vi "rio_veloster8.vi"() -> ()   [LabVIEW 2012]
uses:
  <vilib>/xnet/xnet.llb/XNET Frame CAN.ctl
  <vilib>/xnet/xnet.llb/XNET Frame Type CAN.ctl
  G_rio.vi
  <vilib>/FPGAPlugInAG/cRIO-9113/niLvFpga_Open_cRIO-9113.vi
  <vilib>/rvi/interface/common/dynamic/niFpgaDynamicAddResources.vi
  <vilib>/FPGAPlugInAG/Dynamic/niLvFpga_Abort_Dynamic.vi
  <vilib>/FPGAPlugInAG/Dynamic/niLvFpga_Run_Dynamic.vi
  <vilib>/Utility/error.llb/Error Cluster From Error Code.vi
  <vilib>/Instr/_visa.llb/VISA Configure Serial Port (Instr).vi
  <vilib>/xnet/xnet.llb/XNET Create Session (Frame Output Stream).vi
  <vilib>/xnet/xnet.llb/XNET Create Session (Frame Input Stream).vi
  <vilib>/xnet/xnet.llb/XNET Read (Frame CAN).vi
  <vilib>/rvi/errors/niLvFpgaAdjustHostInterfaceError.vi
  <vilib>/xnet/xnet.llb/XNET Write (Frame CAN).vi
  <vilib>/Analysis/Matrix/Numeric/Conversions/Array To Matrix - RA2.vi
  <vilib>/Analysis/Matrix/Numeric/Multiply/Multiply - RM,RM.vi
  <vilib>/Analysis/Matrix/Numeric/Add/Add - RM,RM.vi
  <vilib>/Analysis/baseanly.llb/Real Inverse Matrix.vi
  <vilib>/Analysis/Matrix/Numeric/Subtract/Subtract - RM,RM.vi
  <vilib>/Analysis/Matrix/Numeric/Conversions/Array To Matrix - RA.vi
  <vilib>/Analysis/Matrix/Numeric/Multiply/Multiply - R,RM.vi
  <vilib>/Analysis/Matrix/Numeric/Conversions/Matrix To Array - RM.vi
  <vilib>/rvi/interface/nirviOpenFPGA/nirviOpenFPGA.xnode
  FPGA Bitfiles/autonomous_FPGATarget2_fpga3_8ngZXtRRx8Y.lvbitx
  fpga/fpga3.vi
  <vilib>/rvi/interface/nirviMethod/nirviMethod.xnode
  <vilib>/rvi/interface/nirviReadWriteControl/nirviReadWriteControl.xnode
  <vilib>/rvi/interface/Simulation/niFpgaSimulationCallBeginRW.vi
  <vilib>/FPGAPlugInAG/Dynamic/niLvFpga_StartFifo_Dynamic.vi
  <vilib>/rvi/errors/niLvFpgaMergeErrorWithErrorCode.vi
  <resource>/objmgr/xnet.rc
  NiFpgaLv.dll
  <vilib>/FPGAPlugInAG/Dynamic/niLvFpga_ReadFifo_Dynamic.vi
  <vilib>/Analysis/Matrix/NI_Matrix.lvlib
  <vilib>/Analysis/NI_AALBase.lvlib
panel:
  out "Pos_time 10":i32
  out "FPGA VI Reference Out":refnum<k20>
  out "T PWM":u16
  out "B PWM":u16
  out "solenoid":bool
  out "brk enc":u8
  out "shift lever":dbl
  in  "LCM":bool=TRUE
  out "mobileye":u8[](array[numeric])
  out "timer":u32
  out "Mobileye_time 100":u32
  out "H_GPS":dbl
  out "pos":dbl[](array[numeric])
  out "gps pos error":dbl
  in  "GPS init":bool=TRUE
  out "battery voltage":dbl
  in  "Gear Manual":i32(slide)=1 scale=-1.0..1.0
  out "map":i32=2
  out "P, R, D":i32
  out "kalman heading error":dbl
  out "Kalman init":bool
  out "VS_CAN":dbl
  in  "brake":bool
  in  "Slide":dbl(slide) min=-50.0 max=50.0 step=50.0 scale=-50.0..50.0
  out "novatel":refnum<visa-resource-name>
  in  "ublox":bool=TRUE
  out "rest":u8[](array[numeric])
  out "GPS_novatel_time":u32
  out "GPS_Ublox_time 100":u32
  out "Con_time 10":i32
  out "CAN_time 10":u32
  out "gps2":refnum<visa-resource-name>
  out "gps1":refnum<visa-resource-name>
  out "Heading":dbl
  out "ecef ref":dbl[](array[numeric])
  out "h_gps":dbl
  out "pos_gps":dbl[](array[numeric]) format="%#_19f"
  out "get heading":bool
  out "get position":bool
  out "dt":dbl
  out "rt":dbl
  out "CAN Comm Enabled":bool
  in  "SPAS Enable":bool=TRUE
  in  "file write":bool
  out "data write":refnum<file>
  out "file rw error":errorcluster
  out "car can error":errorcluster
  out "CAN write":refnum<k21>
  out "CAN read":refnum<k21>
  out "Ref steer":dbl=1.0
  in  "Steer input":bool=TRUE
  in  "Ref steer manual":dbl(knob) scale=-550.0..550.0
  out "Ref vel":dbl=1.0
  in  "Ref vel manual":dbl
  in  "Velocity input":bool
  out "Auto":bool
  out "Run":bool
  out "E - STOP":bool
  out "Throttle Enable":bool=TRUE
  # "P"
  # "R"
  # "D"
  # "Ref steer manual"
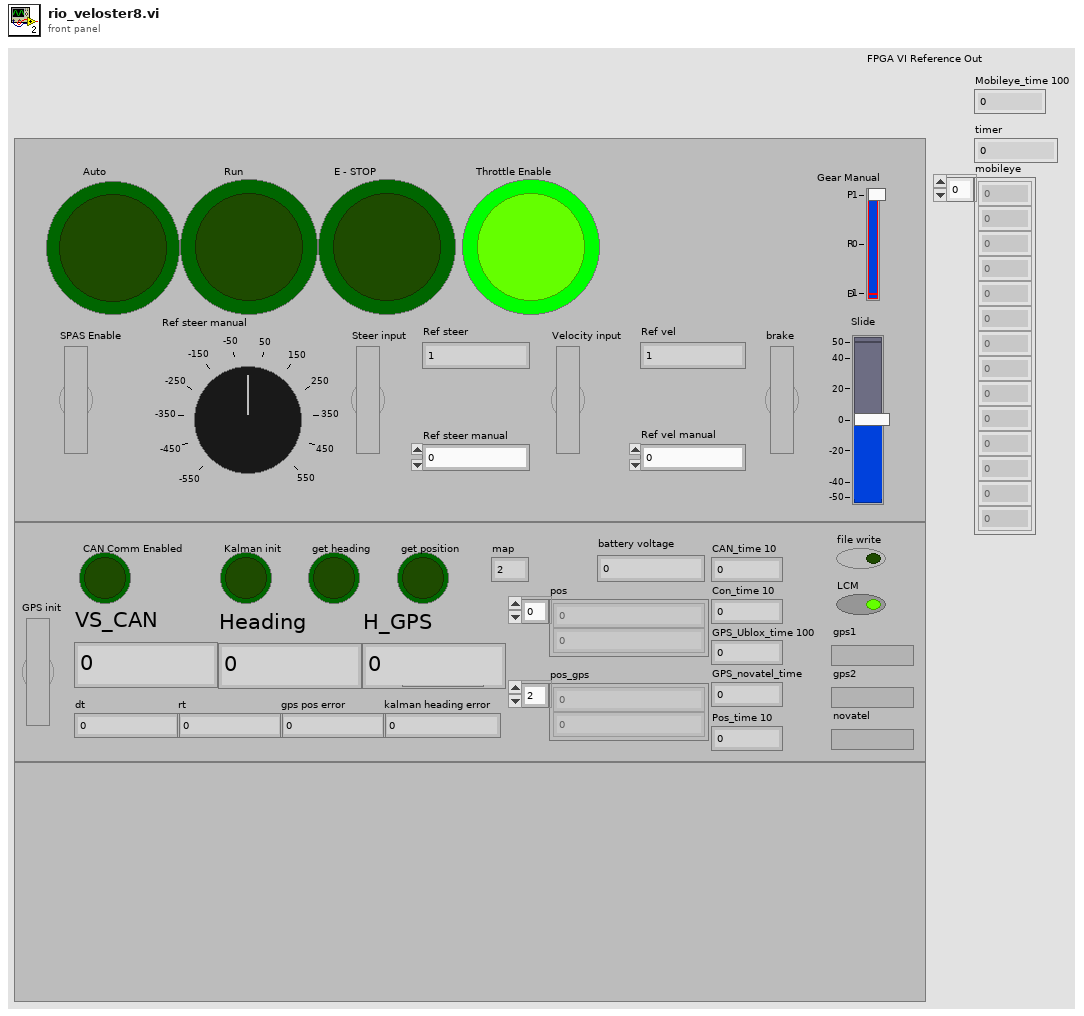
[diagram p1: front panel]
types:
  T1 = enum16{"open", "replace", "create", "open or create", "replace or create", "replace or create with confirmation"}
  T2 = typedef "XNET Frame CAN.ctl" = cluster{"timestamp":timestamp, "payload":u8[], "identifier":u32, "type":T3, "extended?":bool, "echo?":bool}
  T3 = typedef "XNET Frame Type CAN.ctl" = u8
  T4 = cluster{"connection ID":refnum<k16>, "net address":u32, "port":u16}
  T5 = cluster{"hash":i64, "sys time":i64, "mobileye":u8[]}
  T6 = cluster{"hash":i64, "sys time":i64, "time":dbl, "yaw_rate":dbl, "mdps torque":dbl, "mdps str_ang":dbl, "VS_CAN":dbl, "lat_accel":dbl, "mcp":dbl, "accel pedal value":dbl, "tps":dbl, "odometer":dbl, "battery voltage":dbl, "WHL_SPD_RR":dbl, "WHL_SPD_RL":dbl, "WHL_SPD_FR":dbl, "WHL_SPD_FL":dbl}
  T7 = cluster{"LCC[0]":dbl, "LCC[1]":dbl, "LCC[2]":dbl, "LCC[3]":dbl, "LCC[4]":dbl, "LCC[5]":dbl, "LCC[6]":dbl, "LCC[7]":dbl, "LCC[8]":dbl, "LCC[9]":dbl, "LCC[10]":dbl, "LCC[11]":dbl, "LCC[12]":dbl, "LCC[13]":dbl, "LCC[14]":dbl}
  T8 = cluster{"hash":i64, "sys time":i64, "time":dbl, "x":dbl, "y":dbl, "h":dbl, "numSV":i32, "postype":i32, "lag":i32, "hordev":dbl, "lat":dbl, "lon":dbl, "hgt":dbl, "map_idx":i32}
  T9 = cluster{"vel[0]":dbl, "vel[1]":dbl, "vel[2]":dbl, "vel[3]":dbl, "vel[4]":dbl, "vel[5]":dbl, "vel[6]":dbl}
  T10 = cluster{"hash":i64, "sys time":i64, "time":dbl, "speed":dbl, "heading":dbl, "lat":dbl, "lon":dbl}
  T11 = cluster{"output[0]":dbl, "output[1]":dbl, "output[2]":dbl, "output[3]":dbl, "output[4]":dbl, "output[5]":dbl, "output[6]":dbl, "output[7]":dbl, "output[8]":dbl, "output[9]":dbl, "output[10]":dbl, "output[11]":dbl, "output[12]":dbl, "output[13]":dbl, "output[14]":dbl}
  T12 = cluster{"output[0]":dbl, "output[1]":dbl, "output[2]":dbl, "output[3]":dbl, "output[4]":dbl, "output[5]":dbl, "output[6]":dbl}
  T13 = typedef "NI_Matrix.lvlib/RealMatrix.ctl" = dbl[][]
  T14 = cluster{"Real 2D Array[0]":dbl, "Real 2D Array[1]":dbl, "Real 2D Array[2]":dbl, "Real 2D Array[3]":dbl, "Real 2D Array[4]":dbl}
  T15 = cluster{"hash":i64, "sys time":i64, "dt":dbl, "x":dbl, "y":dbl, "speed":dbl, "heading":dbl, "yaw_rate":dbl}
  T16 = cluster{"hash":i64, "sys time":i64, "ref_vel":dbl, "ref_steer":dbl}
  T17 = cluster{"hash":i64, "sys time":i64, "Auto":bool, "Run":bool, "Solenoid":bool, "T lim":bool, "brk_enc":u8, "B PWM":u16, "T PWM":u16, "ref_vel":dbl, "ref_bkr_enc":dbl, "ref_apv":dbl, "ref_steer":dbl}
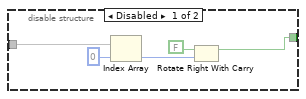
[diagram p5: hidden frame]
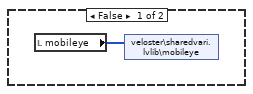
[diagram p7: hidden frame]
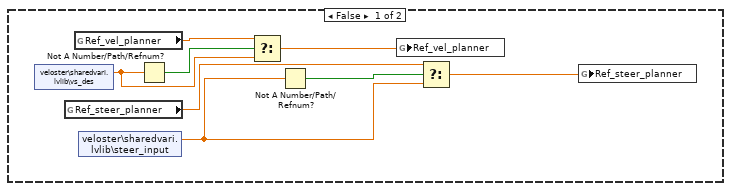
[diagram p9: hidden frame]
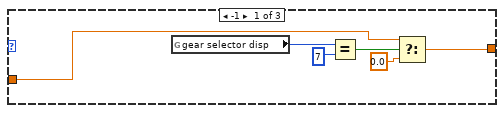
[diagram p14: hidden frame]
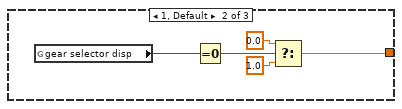
[diagram p18: hidden frame]
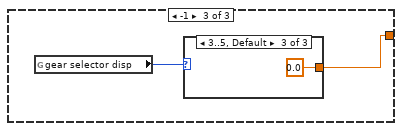
[diagram p19: hidden frame]
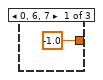
[diagram p20: hidden frame]
diagram:
  n1 = flat-sequence {
    frame #0 {
      w3 = FALSE ("GPS init")
      w2 = 0.0 ("Ref_vel_planner")
      n2 = xnode "Open FPGA VI Reference"() -> ("FPGA VI Reference Out"=w12:refnum<k20>, "error out"=w11:errorcluster)  [unwired: 2 in]
      n3 = global write "G_rio.vi" "Ref_steer_planner"(w2) -> ()
      n4 = global write "G_rio.vi" "Ref_vel_planner"(w2) -> ()
      n5 = local write "rest"(u8[] [] ("rest")) -> ()
      n6 = local write "brake"(w3) -> ()
      n7 = local write "GPS init"(w3) -> ()
      n8 = local write "Velocity input"(w3) -> ()
      n9 = xnode "Invoke Method"("FPGA VI Reference In"=w12, "error in"=w11) -> ("FPGA VI Reference Out"=w10:refnum<k20>, "error out"=w9:errorcluster)
      n10 = xnode "Invoke Method"("FPGA VI Reference In"=w10, "error in"=w9, "Wait Until Done (F)"=FALSE) -> ("FPGA VI Reference Out"=w8:refnum<k20>, "error out"=w7:errorcluster)
      n11 = xnode "Invoke Method"("FPGA VI Reference In"=w8, "error in"=w7) -> ("FPGA VI Reference Out"=w6:refnum<k20>, "error out"=w5:errorcluster)
      n12 = xnode "Invoke Method"("FPGA VI Reference In"=w6, "error in"=w5) -> ("FPGA VI Reference Out"=→"FPGA VI Reference Out":refnum<k20>)  [unwired: 1 out]
    }
    frame #1 {
      n13 = flat-sequence {
        frame #0 {
          w61 = 9 ("map")
          n14 = global write "G_rio.vi" "T lim counter 2"(u16 300 ("T lim counter 2")) -> ()
          n15 = local write "rest"(u8[] [] ("rest")) -> ()
          n16 = call "getecefdcmref.vi"("map"=w61) -> ("XYZ"=→"ecef ref":dbl[])  [unwired: 10 in, 4 out]
          "Kalman init" <- TRUE ("pos linit")
          "map" <- w61
        }
      }
      n17 = disable-structure shown="Enabled" {
        frame Enabled {
          n18 = call-poly "VISA Configure Serial Port"("VISA resource name"=refnum<visa-resource-name> "ASRL1::INSTR", "timeout (10sec)"=u32 10, "baud rate (9600)"=u32 9600) -> ("VISA resource name out"=→"novatel":refnum<visa-resource-name>)  [unwired: 11 in, 1 out]
          n19 = call-poly "VISA Configure Serial Port"("VISA resource name"=refnum<visa-resource-name> "USB0::0x1546::0x01A6::NI-VISA-1::1::RAW", "timeout (10sec)"=u32 1, "baud rate (9600)"=u32 115200) -> ("VISA resource name out"=→"gps1":refnum<visa-resource-name>)  [unwired: 11 in, 1 out]
          n20 = call-poly "VISA Configure Serial Port"("VISA resource name"=refnum<visa-resource-name> "USB0::0x1546::0x01A6::NI-VISA-0::1::RAW", "timeout (10sec)"=u32 1, "baud rate (9600)"=u32 115200) -> ("VISA resource name out"=→"gps2":refnum<visa-resource-name>)  [unwired: 11 in, 1 out]
        }
        frame Disabled {
        }
      }
      n21 = flat-sequence {
        frame #0 {
          n22 = property class="XNET System"() -> (error out=w28:errorcluster, "Devices"=w42:refnum<k21>[])  [unwired: 2 in, 1 out]
          n23 = Index Array(array=w42, index=0) -> (element=w40:refnum<k21>)
          n24 = property class="XNET Device"(reference=w40, error in=w28) -> (error out=→"car can error":errorcluster, "Intfs"=w39:refnum<k21>[])  [unwired: 1 out]
          n25 = Index Array(array=w39, index=0) -> (element=w30:refnum<k21>)
          n26 = call-poly <vilib>:"XNET Create Session.vi"("cluster (:memory:)"=refnum<k21> "nixnet_example.CAN_Cluster", "interface"=w30) -> ("session out"=w31:refnum<k21>)  [unwired: 1 in, 12 out]
          n27 = call-poly <vilib>:"XNET Create Session.vi"("cluster (:memory:)"=refnum<k21> "nixnet_example.CAN_Cluster", "interface"=w30) -> ("session out"=w37:refnum<k21>)  [unwired: 1 in, 12 out]
          n28 = property class="XNET Session"(reference=w31, "Intf.BaudRate"=u32 500000 ("Interface:Baud Rate")) -> (reference out=w33:refnum<k21>)  [unwired: 1 in, 1 out]
          n29 = property class="XNET Session"(reference=w37, "Intf.BaudRate"=u32 500000 ("Interface:Baud Rate")) -> (reference out=w35:refnum<k21>)  [unwired: 1 in, 1 out]
          n30 = call <vilib>:"XNET Start.vi"("session in"=w33) -> ("session out"=→"CAN read":refnum<k21>)  [unwired: 1 in, 13 out]
          n31 = call <vilib>:"XNET Start.vi"("session in"=w35) -> ("session out"=→"CAN write":refnum<k21>)  [unwired: 1 in, 13 out]
        }
      }
      n32 = case shown="True" "file write" {
        frame False {
        }
        frame True {
          n33 = Open/Create/Replace File(file path (use dialog)=path "c:/datasave", operation (0:open)=T1."replace or create", access (0:read/write)=enum16{"read/write", "read-only", "write-only"}."write-only") -> (refnum out=→"data write":refnum<file>, cancelled=w65:bool, error out=→"file rw error":errorcluster)  [unwired: 3 in]
          n34 = Not(x=w65) -> (.not. x?=w64:bool)
          n35 = local write "file write"(w64) -> ()
        }
      }
      n36 = case shown="True" TRUE {
        frame False {
        }
        frame True {
          n37 = flat-sequence {
            frame #0 {
              w22 = u16 7667 ("port")
              n38 = Decrement(x=w22) -> (x-1=w21:u16)
              n39 = UDP Open(11:w21) -> (port=w24:refnum<k16>)  [unwired: 4 in, 2 out]
              n40 = global read "G_rio.vi" "LCM"() -> (w26:T4)
              n41 = Bundle By Name(cluster=w26, "port"=w22, "connection ID"=w24, "net address"=u32 4294967295) -> (w25:T4)
              n42 = global write "G_rio.vi" "LCM"(w25) -> ()
            }
          }
          n43 = flat-sequence {
            frame #0 {
              w16 = u16 7668 ("port")
              n44 = global read "G_rio.vi" "LCM PC"() -> (w20:T4)
              n45 = UDP Open(11:w16) -> (port=w18:refnum<k16>)  [unwired: 4 in, 2 out]
              n46 = Bundle By Name(cluster=w20, "port"=w16, "connection ID"=w18, "net address"=u32 0) -> (w19:T4)
              n47 = global write "G_rio.vi" "LCM PC"(w19) -> ()
            }
          }
        }
      }
    }
    frame #2 {
      (unwired) FALSE
      n48 = disable-structure shown="Enabled" {
        frame Enabled {
          n49 = while {
            stop <- FALSE stop-if-true
            n50 = flat-sequence {
              frame #0 {
                n51 = Wait Until Next ms Multiple(millisecond multiple=u32 100) -> (millisecond timer value=w71:u32)
                n52 = flat-sequence {
                  tunnel: w71 -> [w73]
                  frame #0 {
                    n53 = feedback #1(w73) -> (w74:u32)
                    n54 = feedback-in #1(w73) -> ()
                    n55 = Subtract(x=w73, y=w74) -> (x-y=→"Mobileye_time 100":u32)
                  }
                }
              }
              frame #1 {
                n56 = local read "FPGA VI Reference Out"() -> (w120:refnum<k20>)
                n57 = xnode "Read/Write Control"("FPGA VI Reference In"=w120) -> ("m 700"=w80:u8[], "m 760"=w116:u8[], "m 710"=w105:u8[], "m 711"=w101:u8[], "m 720"=w99:u8[], "m 721"=w98:u8[], "m 722"=w97:u8[], "m 723"=w96:u8[], "m 724"=w95:u8[], "m 725"=w94:u8[], "m 726"=w93:u8[], "m 727"=w92:u8[], "m 728"=w91:u8[], "m 729"=w90:u8[])  [unwired: 1 in, 2 out]
                n58 = Build Array(w99, w98, w97, w96, w95, w94, w93, w92, w91, w90) -> (w89:u8[][])
                n59 = Index Array(array=w80, index #1=4 ("index"), index #4=8 ("index"), index #5=11 ("index")) -> (element #1=w113:u8, element #2=w112:u8, element #3=w111:u8, element #4=w110:u8, element #5=w109:u8)  [unwired: 2 in]
                n60 = Array Subset(array=w80, index=0, length=4) -> (w77:u8[])
                n61 = Array Subset(array=w116, index=4, length=3) -> (w108:u8[])
                n62 = Array Subset(array=w105, index=5, length=7) -> (w104:u8[])
                n63 = Array Subset(array=w101, index=6, length=6) -> (w100:u8[])
                n64 = Index Array(array=w77, index #1=0 ("index")) -> (element #1=w86:u8, element #2=w85:u8, element #3=w84:u8, element #4=w83:u8)  [unwired: 3 in]
                n65 = Build Array (concatenate)(w77, w113, w112, w111, w110, w109, w108, w104, w100) -> (w88:u8[])
                n66 = Join Numbers(hi=w86, lo=w85) -> ((hi.lo)=w82:u16)
                n67 = Join Numbers(hi=w84, lo=w83) -> ((hi.lo)=w81:u16)
                n68 = for {
                  tunnel: w89 -> [w122] mode=indexing
                  shift-right: [w125] -> w75
                  shift-left: w88 -> [w126]
                  n69 = Array Subset(array=w122, index=4, length=8) -> (w121:u8[])
                  n70 = disable-structure shown="Enabled" {
                    disable-tunnel: [w129 TRUE ("lsb carry out")] -> w127
                    disable-tunnel: w121 -> [w128 _]
                    frame Disabled {
                      n71 = Index Array(array=w128, index=0) -> (element=w131:u8)
                      n72 = Rotate Right With Carry(2:w131, 3:FALSE ("carry")) -> (1:w129:bool)  [unwired: 1 out]
                    }
                    frame Enabled {
                    }
                  }
                  n73 = case shown="True" w127 {
                    tunnel: w126 -> [w134 w137]
                    tunnel: [w134 w136] -> w125
                    tunnel: w121 -> [_ w135]
                    frame False {
                    }
                    frame True {
                      n74 = Build Array (concatenate)(w137, w135) -> (w136:u8[])
                    }
                  }
                }
                "mobileye" <- w75
                n75 = Join Numbers(hi=w82, lo=w81) -> ((hi.lo)=→"timer":u32)
              }
              frame #2 {
                n76 = local read "LCM"() -> (w138:bool)
                n77 = case shown="True" w138 {
                  frame False {
                    n78 = local read "mobileye"() -> (w139:u8[])
                    n79 = shared-variable "veloster\\sharedvari.lvlib\\mobileye"(w139) -> ()  [unwired: 1 in, 1 out]
                  }
                  frame True {
                    n80 = Get Date/Time In Seconds() -> (seconds since 1Jan1904=w144:timestamp)
                    n81 = local read "mobileye"() -> (w145:u8[])
                    n82 = To Double Precision Float(number=w144) -> (double precision float=w143:dbl)
                    n83 = global read "G_rio.vi" "LCM_EYE_RAW_T"() -> (w153:T5)
                    n84 = Unbundle By Name(w153) -> ("hash"=w152:i64)
                    n85 = Multiply(x=w143, y=1000000.0) -> (x*y=w141:dbl)
                    n86 = To Quad Integer(1:w141) -> (0:w140:i64)
                    n87 = call "hash.vi"("input"=w152) -> ("output"=w151:i64)  [unwired: 10 in]
                    n88 = Bundle By Name(cluster=w153, "hash"=w151, "sys time"=w140, "mobileye"=w145) -> (w150:T5)
                    n89 = Flatten To String(anything=w150, prepend array or string size? (T)=FALSE) -> (data string=w148:string)  [unwired: 2 in, 2 out]
                    n90 = global read "G_rio.vi" "LCM"() -> (w149:T4)
                    n91 = call "LCM_send.vi"("DATA"=w148, "ID"="EYE_RAW_T", "LCM"=w149) -> ()  [unwired: 6 in, 3 out]
                  }
                }
              }
            }
          }
        }
        frame Disabled {
        }
      }
      n92 = while {
        stop <- FALSE stop-if-true
        n93 = flat-sequence {
          frame #0 {
            n94 = Wait Until Next ms Multiple(millisecond multiple=u32 10) -> (millisecond timer value=w1396:u32)
            n95 = flat-sequence {
              tunnel: w1396 -> [w1399]
              frame #0 {
                n96 = feedback #2(w1399) -> (w1400:u32)
                n97 = feedback-in #2(w1399) -> ()
                n98 = Subtract(x=w1399, y=w1400) -> (x-y=→"CAN_time 10":u32)
              }
            }
          }
          frame #1 {
            n99 = local read "CAN read"() -> (w1404:refnum<k21>)
            n100 = call-poly <vilib>:"XNET Read.vi"("session in"=w1404) -> ("data"=w1403:T2[])  [unwired: 3 in, 11 out]
            n101 = Empty Array?(array=w1403) -> (empty?=w1402:bool)
            n102 = for {
              tunnel: w1403 -> [w1406] mode=indexing
              n103 = Unbundle By Name(w1406) -> ("timestamp"=w1405:timestamp, "identifier"=w1408:u32, "payload"=w1407:u8[])
              n104 = case shown="220" w1408 {
                tunnel: w1407 -> [_ w1443 w1478 w1497 w1538 w1569 w1601 w1608]
                tunnel: w1405 -> [_ w1438 _ _ _ _ _ _]
                frame 0, Default {
                }
                frame 544 {
                  w1412 = u16 8191
                  w1419 = u16 2047
                  n105 = global write "G_rio.vi" "timestamp"(w1438) -> ()
                  n106 = Index Array(array=w1443, index #1=5 ("index"), index #2=4 ("index"), index #3=1 ("index"), index #4=0 ("index"), index #5=7 ("index"), index #6=6 ("index")) -> (element #1=w1435:u8, element #2=w1434:u8, element #3=w1433:u8, element #4=w1432:u8, element #5=w1431:u8, element #6=w1430:u8)
                  n107 = Join Numbers(hi=w1433, lo=w1432) -> ((hi.lo)=w1420:u16)
                  n108 = Join Numbers(hi=w1431, lo=w1430) -> ((hi.lo)=w1411:u16)
                  n109 = And(x=w1435, y=u8 15) -> (x .and. y?=w1428:u8)
                  n110 = Logical Shift(y=i16 -6, x=w1433) -> (x << y=w1422:u8)
                  n111 = Logical Shift(y=i16 -6, x=w1431) -> (x << y=w1415:u8)
                  n112 = Join Numbers(hi=w1428, lo=w1434) -> ((hi.lo)=w1425:u16)
                  n113 = Equal To 0?(x=w1422) -> (x = 0?=w1423:bool)
                  n114 = And(x=w1419, y=w1420) -> (x .and. y?=w1418:u16)
                  n115 = And(x=w1412, y=w1411) -> (x .and. y?=w1410:u16)
                  n116 = Not Equal?(x=w1419, y=w1418) -> (x != y?=w1424:bool)
                  n117 = Not Equal?(x=w1412, y=w1410) -> (x != y?=w1413:bool)
                  n118 = Equal To 0?(x=w1415) -> (x = 0?=w1414:bool)
                  n119 = Not Equal?(x=u16 4095, y=w1425) -> (x != y?=w1426:bool)
                  n120 = case shown="True" w1426 {
                    tunnel: w1425 -> [_ w1466]
                    frame False {
                    }
                    frame True {
                      n121 = global write "G_rio.vi" "mcp"(w1466) -> ()
                      n122 = To Double Precision Float(number=w1466) -> (double precision float=w1468:dbl)
                      n123 = Greater?(x=w1466, y=u16 10) -> (0:w1465:bool)
                      n124 = global write "G_rio.vi" "brake_act_can"(w1465) -> ()
                      n125 = Multiply(x=w1468, y=10.0) -> (x*y=w1463:dbl)
                      n126 = Square Root(x=w1463) -> (sqrt(x)=w1462:dbl)
                      n127 = global write "G_rio.vi" "Brake Encoder mcp"(w1462) -> ()
                    }
                  }
                  n128 = And(x=w1423, y=w1424) -> (x .and. y?=w1417:bool)
                  n129 = And(x=w1414, y=w1413) -> (x .and. y?=w1409:bool)
                  n130 = case shown="True" w1417 {
                    tunnel: w1418 -> [_ w1461]
                    frame False {
                    }
                    frame True {
                      n131 = To Double Precision Float(number=w1461) -> (double precision float=w1460:dbl)
                      n132 = Multiply(x=w1460, y=0.01) -> (x*y=w1458:dbl)
                      n133 = Subtract(x=w1458, y=10.23) -> (x-y=w1456:dbl)
                      n134 = global write "G_rio.vi" "lat_accel"(w1456) -> ()
                    }
                  }
                  n135 = case shown="True" w1409 {
                    tunnel: w1410 -> [_ w1455]
                    frame False {
                    }
                    frame True {
                      n136 = To Double Precision Float(number=w1455) -> (double precision float=w1454:dbl)
                      n137 = Multiply(x=w1454, y=0.01) -> (x*y=w1452:dbl)
                      n138 = Subtract(x=w1452, y=40.95) -> (x-y=w1445:dbl)
                      n139 = Add(x=w1445, y=-0.034) -> (x+y=w1444:dbl)
                      n140 = Multiply(x=w1444, y=1.045) -> (x*y=w1448:dbl)
                      n141 = Add(x=w1448, y=0.0) -> (x+y=w1447:dbl)
                      n142 = global write "G_rio.vi" "yaw_rate"(w1447) -> ()
                    }
                  }
                }
                frame 809 {
                  # "10ms"
                  n143 = Index Array(array=w1478, index #1=5 ("index"), index #2=6 ("index"), index #3=4 ("index")) -> (element #1=w1475:u8, element #2=w1472:u8)  [unwired: 1 out]
                  n144 = Not Equal?(x=w1475, y=u8 255 ("x")) -> (x != y?=w1471:bool)
                  n145 = Not Equal?(x=w1472, y=u8 255 ("x")) -> (x != y?=w1470:bool)
                  n146 = case shown="True" w1471 {
                    tunnel: w1475 -> [_ w1490]
                    frame False {
                    }
                    frame True {
                      n147 = Subtract(x=w1490, y=u8 32) -> (x-y=w1488:u8)
                      n148 = To Double Precision Float(number=w1488) -> (double precision float=w1487:dbl)
                      n149 = Multiply(x=w1487, y=100.0) -> (x*y=w1485:dbl)
                      n150 = Divide(x=w1485, y=213.0) -> (x/y=w1483:dbl)
                      n151 = global write "G_rio.vi" "tps"(w1483) -> ()
                    }
                  }
                  n152 = case shown="True" w1470 {
                    tunnel: w1472 -> [_ w1482]
                    frame False {
                    }
                    frame True {
                      n153 = To Double Precision Float(number=w1482) -> (double precision float=w1481:dbl)
                      n154 = Multiply(x=w1481, y=0.3906) -> (x*y=w1480:dbl)
                      n155 = global write "G_rio.vi" "accel pedal value"(w1480) -> ()
                    }
                  }
                }
                frame 914 {
                  # "20ms"
                  n156 = Array Subset(array=w1497, index=0, length=7) -> (w1494:u8[])
                  n157 = Index Array(array=w1497, index #1=7 ("index"), index #2=2 ("index"), index #3=1 ("index"), index #4=4 ("index"), index #5=3 ("index")) -> (element #1=w1491:u8, element #2=w1503:u8, element #3=w1502:u8, element #4=w1499:u8, element #5=w1498:u8)
                  n158 = Add Array Elements(numeric array=w1494) -> (sum=w1492:u8)
                  n159 = Equal?(x=w1492, y=w1491) -> (x = y?=w1493:bool)
                  n160 = case shown="True" w1493 {
                    tunnel: w1503 -> [_ w1517]
                    tunnel: w1502 -> [_ w1516]
                    tunnel: w1499 -> [_ w1513]
                    tunnel: w1498 -> [_ w1512]
                    frame False {
                    }
                    frame True {
                      w1508 = u16 4095 ("y")
                      n161 = Join Numbers(hi=w1517, lo=w1516) -> ((hi.lo)=w1509:u16)
                      n162 = Join Numbers(hi=w1513, lo=w1512) -> ((hi.lo)=w1514:u16)
                      n163 = Not Equal?(x=w1514, y=u16 32767 ("x")) -> (x != y?=w1510:bool)
                      n164 = And(x=w1508, y=w1509) -> (x .and. y?=w1507:u16)
                      n165 = Not Equal?(x=w1508, y=w1507) -> (x != y?=w1511:bool)
                      n166 = case shown="True" w1511 {
                        tunnel: w1507 -> [_ w1529]
                        frame False {
                        }
                        frame True {
                          n167 = To Double Precision Float(number=w1529) -> (double precision float=w1528:dbl)
                          n168 = Subtract(x=w1528, y=2048.0) -> (x-y=w1527:dbl)
                          n169 = Multiply(x=w1527, y=0.01) -> (x*y=w1530:dbl)
                          n170 = global write "G_rio.vi" "mdps torque"(w1530) -> ()
                        }
                      }
                      n171 = case shown="True" w1510 {
                        tunnel: w1514 -> [_ w1524]
                        frame False {
                        }
                        frame True {
                          n172 = To Double Precision Float(number=w1524) -> (double precision float=w1521:dbl)
                          n173 = Subtract(x=w1521, y=65536.0) -> (x-y=w1522:dbl)
                          n174 = Greater?(x=w1521, y=32767.0 ("x")) -> (0:w1525:bool)
                          n175 = Select(t=w1522, s=w1525, f=w1521) -> (s? t:f=w1520:dbl)
                          n176 = Multiply(x=w1520, y=0.1) -> (x*y=w1518:dbl)
                          n177 = global write "G_rio.vi" "mdps str_ang"(w1518) -> ()
                        }
                      }
                    }
                  }
                }
                frame 1087 {
                  w1535 = u8 15 ("y")
                  # "10ms"
                  n178 = Index Array(array=w1538, index=1) -> (element=w1536:u8)
                  n179 = And(x=w1536, y=w1535) -> (x .and. y?=w1534:u8)
                  n180 = Not Equal?(x=w1534, y=w1535) -> (x != y?=w1533:bool)
                  n181 = case shown="True" w1533 {
                    tunnel: w1534 -> [_ w1539]
                    frame False {
                    }
                    frame True {
                      n182 = global write "G_rio.vi" "gear selector disp"(w1539) -> ()
                    }
                  }
                }
                frame 1200 {
                  w1543 = u16 16383 ("x")
                  w1556 = u16 16383 ("x")
                  # "20ms"
                  n183 = Index Array(array=w1569, index #1=1 ("index"), index #2=0 ("index"), index #3=3 ("index"), index #4=2 ("index"), index #5=5 ("index"), index #6=4 ("index"), index #7=7 ("index"), index #8=6 ("index")) -> (element #1=w1548:u8, element #2=w1547:u8, element #3=w1546:u8, element #4=w1545:u8, element #5=w1566:u8, element #6=w1565:u8, element #7=w1561:u8, element #8=w1560:u8)
                  n184 = Join Numbers(hi=w1548, lo=w1547) -> ((hi.lo)=w1544:u16)
                  n185 = Join Numbers(hi=w1546, lo=w1545) -> ((hi.lo)=w1542:u16)
                  n186 = Join Numbers(hi=w1566, lo=w1565) -> ((hi.lo)=w1564:u16)
                  n187 = Join Numbers(hi=w1561, lo=w1560) -> ((hi.lo)=w1557:u16)
                  n188 = And(x=w1544, y=w1543) -> (x .and. y?=w1541:u16)
                  n189 = And(x=w1543, y=w1542) -> (x .and. y?=w1540:u16)
                  n190 = And(x=w1564, y=w1556) -> (x .and. y?=w1555:u16)
                  n191 = And(x=w1556, y=w1557) -> (x .and. y?=w1554:u16)
                  n192 = Not Equal?(x=w1555, y=w1556) -> (x != y?=w1559:bool)
                  n193 = Not Equal?(x=w1556, y=w1554) -> (x != y?=w1558:bool)
                  n194 = And(x=w1559, y=w1558) -> (x .and. y?=w1553:bool)
                  n195 = case shown="True" w1553 {
                    tunnel: w1555 -> [_ w1588]
                    tunnel: w1554 -> [_ w1587]
                    tunnel: w1541 -> [_ w1580]
                    tunnel: w1540 -> [_ w1579]
                    frame False {
                    }
                    frame True {
                      w1575 = 0.03125 ("y")
                      w1586 = 0.03125 ("y")
                      n196 = To Double Precision Float(number=w1580) -> (double precision float=w1577:dbl)
                      n197 = To Double Precision Float(number=w1579) -> (double precision float=w1574:dbl)
                      n198 = To Double Precision Float(number=w1588) -> (double precision float=w1578:dbl)
                      n199 = To Double Precision Float(number=w1587) -> (double precision float=w1571:dbl)
                      n200 = Multiply(x=w1577, y=w1575) -> (x*y=w1576:dbl)
                      n201 = Multiply(x=w1575, y=w1574) -> (x*y=w1573:dbl)
                      n202 = Multiply(x=w1578, y=w1586) -> (x*y=w1572:dbl)
                      n203 = Multiply(x=w1586, y=w1571) -> (x*y=w1570:dbl)
                      n204 = global write "G_rio.vi" "WHL_SPD_FL"(w1576) -> ()
                      n205 = global write "G_rio.vi" "WHL_SPD_FR"(w1573) -> ()
                      n206 = global write "G_rio.vi" "WHL_SPD_RL"(w1572) -> ()
                      n207 = Add(x=w1572, y=w1570) -> (x+y=w1585:dbl)
                      n208 = global write "G_rio.vi" "WHL_SPD_RR"(w1570) -> ()
                      n209 = Multiply(x=w1585, y=0.5) -> (x*y=w1582:dbl)
                      n210 = Multiply(x=w1582, y=1.028) -> (x*y=w1581:dbl)
                      n211 = global write "G_rio.vi" "vs_esc"(w1581) -> ()
                    }
                  }
                }
                frame 1264 {
                  # "20 ms"
                  n212 = Index Array(array=w1601, index #1=7 ("index"), index #2=6 ("index"), index #3=5 ("index")) -> (element #1=w1595:u8, element #2=w1597:u8, element #3=w1596:u8)
                  n213 = Join Numbers(hi=w1597, lo=w1596) -> ((hi.lo)=w1592:u16)
                  n214 = Join Numbers(hi=u8 0, lo=w1595) -> ((hi.lo)=w1593:u16)
                  n215 = Join Numbers(hi=w1593, lo=w1592) -> ((hi.lo)=w1590:u32)
                  n216 = Not Equal?(x=u32 16777215, y=w1590) -> (x != y?=w1589:bool)
                  n217 = case shown="True" w1589 {
                    tunnel: w1590 -> [_ w1603]
                    frame False {
                    }
                    frame True {
                      n218 = To Double Precision Float(number=w1603) -> (double precision float=w1602:dbl)
                      n219 = global write "G_rio.vi" "odometer"(w1602) -> ()
                    }
                  }
                }
                frame 1349 {
                  # "10 ms"
                  n220 = Index Array(array=w1608, index=3) -> (element=w1606:u8)
                  n221 = Not Equal?(x=w1606, y=u8 255 ("x")) -> (x != y?=w1604:bool)
                  n222 = case shown="True" w1604 {
                    tunnel: w1606 -> [_ w1614]
                    frame False {
                    }
                    frame True {
                      n223 = To Double Precision Float(number=w1614) -> (double precision float=w1613:dbl)
                      n224 = Multiply(x=26.0, y=w1613) -> (x*y=w1611:dbl)
                      n225 = Divide(x=w1611, y=256.0) -> (x/y=w1609:dbl)
                      "battery voltage" <- w1609
                      n226 = global write "G_rio.vi" "battery voltage"(w1609) -> ()
                    }
                  }
                }
              }
            }
            n227 = Not(x=w1402) -> (.not. x?=→"CAN Comm Enabled":bool)
          }
          frame #2 {
            n228 = global read "G_rio.vi" "vs_esc"() -> (w1615:dbl)
            n229 = global read "G_rio.vi" "gear selector disp"() -> (w1619:u8)
            n230 = Negate(x=w1615) -> (-x=w1617:dbl)
            n231 = Equal?(x=w1619, y=u8 7) -> (x = y?=w1618:bool)
            n232 = Select(t=w1617, s=w1618, f=w1615) -> (s? t:f=w1616:dbl)
            "VS_CAN" <- w1616
            n233 = global write "G_rio.vi" "VS_CAN"(w1616) -> ()
          }
          frame #3 {
            n234 = local read "CAN Comm Enabled"() -> (w1622:bool)
            n235 = local read "LCM"() -> (w1623:bool)
            n236 = And(x=w1623, y=w1622) -> (x .and. y?=w1621:bool)
            n237 = case shown="True" w1621 {
              frame False {
              }
              frame True {
                n238 = global read "G_rio.vi" "mcp"() -> (w1650:u16)
                n239 = Get Date/Time In Seconds() -> (seconds since 1Jan1904=w1632:timestamp)
                n240 = global read "G_rio.vi" "timestamp"() -> (w1651:timestamp)
                n241 = global read "G_rio.vi" "odometer"() -> (w1636:dbl)
                n242 = global read "G_rio.vi" "yaw_rate"() -> (w1645:dbl)
                n243 = global read "G_rio.vi" "lat_accel"() -> (w1642:dbl)
                n244 = global read "G_rio.vi" "VS_CAN"() -> (w1637:dbl)
                n245 = To Double Precision Float(number=w1632) -> (double precision float=w1631:dbl)
                n246 = To Double Precision Float(number=w1650) -> (double precision float=w1641:dbl)
                n247 = global read "G_rio.vi" "accel pedal value"() -> (w1639:dbl)
                n248 = global read "G_rio.vi" "battery voltage"() -> (w1638:dbl)
                n249 = global read "G_rio.vi" "mdps str_ang"() -> (w1643:dbl)
                n250 = global read "G_rio.vi" "WHL_SPD_RR"() -> (w1627:dbl)
                n251 = global read "G_rio.vi" "WHL_SPD_RL"() -> (w1626:dbl)
                n252 = global read "G_rio.vi" "WHL_SPD_FR"() -> (w1625:dbl)
                n253 = global read "G_rio.vi" "mdps torque"() -> (w1644:dbl)
                n254 = global read "G_rio.vi" "WHL_SPD_FL"() -> (w1624:dbl)
                n255 = global read "G_rio.vi" "LCM_CAN_T"() -> (w1649:T6)
                n256 = To Double Precision Float(number=w1651) -> (double precision float=w1646:dbl)
                n257 = Unbundle By Name(w1649) -> ("hash"=w1648:i64)
                n258 = Multiply(x=w1631, y=1000000.0) -> (x*y=w1629:dbl)
                n259 = To Quad Integer(1:w1629) -> (0:w1628:i64)
                n260 = call "hash.vi"("input"=w1648) -> ("output"=w1647:i64)  [unwired: 10 in]
                n261 = global read "G_rio.vi" "tps"() -> (w1640:dbl)
                n262 = Bundle By Name(cluster=w1649, "hash"=w1647, "sys time"=w1628, "time"=w1646, "yaw_rate"=w1645, "mdps torque"=w1644, "mdps str_ang"=w1643, "VS_CAN"=w1637, "lat_accel"=w1642, "mcp"=w1641, "accel pedal value"=w1639, "tps"=w1640, "odometer"=w1636, "battery voltage"=w1638, "WHL_SPD_RR"=w1627, "WHL_SPD_RL"=w1626, "WHL_SPD_FR"=w1625, "WHL_SPD_FL"=w1624) -> (w1635:T6)
                n263 = Flatten To String(anything=w1635, prepend array or string size? (T)=FALSE) -> (data string=w1634:string)  [unwired: 2 in, 2 out]
                n264 = disable-structure shown="Enabled" {
                  disable-tunnel: w1634 -> [w1653 _]
                  frame Enabled {
                    n265 = global read "G_rio.vi" "LCM"() -> (w1654:T4)
                    n266 = call "LCM_send.vi"("DATA"=w1653, "ID"="CAN_T", "LCM"=w1654) -> ()  [unwired: 6 in, 3 out]
                  }
                  frame Disabled {
                  }
                }
              }
            }
          }
        }
      }
      n267 = disable-structure shown="Enabled" {
        frame Enabled {
          n268 = disable-structure shown="Enabled" {
            frame Disabled {
              n269 = while {
                stop <- FALSE stop-if-true
                n270 = flat-sequence {
                  frame #0 {
                    n271 = Wait Until Next ms Multiple(millisecond multiple=u32 50) -> ()  [unwired: 1 out]
                  }
                  frame #1 {
                    n272 = local read "FPGA VI Reference Out"() -> (w533:refnum<k20>)
                    n273 = xnode "Read/Write Control"("FPGA VI Reference In"=w533) -> ("FPGA VI Reference Out"=w531:refnum<k20>, "Connection error GPS 1"=w532:bool)  [unwired: 1 in, 1 out]
                    n274 = case shown="False" w532 {
                      tunnel: w531 -> [w535 w655]
                      frame False {
                        n275 = flat-sequence {
                          tunnel: w535 -> [w537]
                          tunnel: [w536] -> w534
                          tunnel: w534 -> [w556]
                          frame #0 {
                            n276 = while {
                              tunnel: w537 -> [w541]
                              tunnel: [w539] -> w536
                              stop <- w540 stop-if-true
                              n277 = flat-sequence {
                                tunnel: w541 -> [w543]
                                tunnel: [w543] -> w538
                                tunnel: [w546] -> w540
                                tunnel: [w545] -> w539
                                tunnel: w538 -> [w552]
                                frame #0 {
                                n278 = Wait Until Next ms Multiple(millisecond multiple=u32 20) -> ()  [unwired: 1 out]
                                }
                                frame #1 {
                                n279 = xnode "Invoke Method"("FPGA VI Reference In"=w552, "Number of Elements"=u32 1, "Timeout (ms)"=1) -> ("FPGA VI Reference Out"=w545:refnum<k20>, "Data"=w547:u8[])  [unwired: 1 in, 2 out]
                                n280 = Index Array(array=w547, index=0) -> (element=w549:u8)
                                n281 = Equal?(x=w549, y=u8 170) -> (x = y?=w546:bool)
                                }
                              }
                            }
                          }
                          frame #1 {
                            w557 = u32 3 ("Number of Elements")
                            n282 = xnode "Invoke Method"("FPGA VI Reference In"=w556, "Number of Elements"=w557, "Timeout (ms)"=w557) -> ("FPGA VI Reference Out"=w555:refnum<k20>, "Data"=w559:u8[], "Elements Remaining"=w553:u32)  [unwired: 1 in, 1 out]
                            n283 = Equal?(x=w559, y=u8[] [68, 18, 28]) -> (x = y?=w560:bool[])
                            n284 = And Array Elements(Boolean array=w560) -> (logical AND=w554:bool)
                            n285 = case shown="True" w554 {
                              tunnel: w555 -> [w563 w568]
                              tunnel: w553 -> [w562 _]
                              frame False {
                                n286 = xnode "Invoke Method"("FPGA VI Reference In"=w563, "Number of Elements"=w562, "Timeout (ms)"=1) -> ()  [unwired: 1 in, 4 out]
                              }
                              frame True {
                                w564 = u32 8 ("Number of Elements")
                                n287 = xnode "Invoke Method"("FPGA VI Reference In"=w568, "Number of Elements"=w564, "Timeout (ms)"=w564) -> ("FPGA VI Reference Out"=w581:refnum<k20>, "error out"=w582:errorcluster, "Data"=w584:u8[])  [unwired: 1 in, 1 out]
                                n288 = Index Array(array=w584, index #1=1 ("index"), index #2=0 ("index"), index #3=5 ("index"), index #4=4 ("index")) -> (element #1=w571:u8, element #2=w572:u8, element #3=w576:u8, element #4=w577:u8)
                                n289 = Join Numbers(hi=w571, lo=w572) -> ((hi.lo)=w573:u16)
                                n290 = Join Numbers(hi=w576, lo=w577) -> ((hi.lo)=w578:u16)
                                n291 = Add(x=w578, y=u16 20) -> (x+y=w580:u16)
                                n292 = xnode "Invoke Method"("FPGA VI Reference In"=w581, "error in"=w582, "Number of Elements"=w580, "Timeout (ms)"=10) -> ("Data"=w566:u8[])  [unwired: 3 out]
                                n293 = Empty Array?(array=w566) -> (empty?=w565:bool)
                                n294 = Build Array (concatenate)(u8[] [170, 68, 18, 28], w584, w566) -> (w585:u8[])
                                n295 = case shown="False" w565 {
                                tunnel: w585 -> [w587 _]
                                tunnel: w573 -> [w586 _]
                                frame False {
                                n296 = case shown="99" w586 {
                                tunnel: w587 -> [_ w590 w628]
                                frame 0, Default {
                                }
                                frame 42 {
                                n297 = local read "ecef ref"() -> (w589:dbl[])
                                n298 = call "novatel_bestpos.vi"("ecef ref"=w589, "gps_data"=w590) -> ("LCC"=w588:dbl[])  [unwired: 9 in]
                                n299 = flat-sequence {
                                tunnel: w588 -> [w593]
                                frame #0 {
                                n300 = Index Array(array=w593, index=1) -> (element=w596:dbl)
                                n301 = Not Equal To 0?(x=w596) -> (x != 0?=w592:bool)
                                n302 = local read "LCM"() -> (w595:bool)
                                n303 = And(x=w592, y=w595) -> (x .and. y?=w591:bool)
                                n304 = case shown="True" w591 {
                                tunnel: w593 -> [_ w616]
                                frame False {
                                }
                                frame True {
                                n305 = Array To Cluster(array=w616) -> (cluster=w624:T7)
                                n306 = Get Date/Time In Seconds() -> (seconds since 1Jan1904=w601:timestamp)
                                n307 = To Double Precision Float(number=w601) -> (double precision float=w600:dbl)
                                n308 = Unbundle(w624) -> ("LCC[0]"=w626:dbl, "LCC[2]"=w615:dbl, "LCC[3]"=w614:dbl, "LCC[4]"=w613:dbl, "LCC[6]"=w612:dbl, "LCC[7]"=w610:dbl, "LCC[8]"=w608:dbl, "LCC[9]"=w606:dbl, "LCC[12]"=w605:dbl, "LCC[13]"=w604:dbl, "LCC[14]"=w603:dbl)  [unwired: 4 out]
                                n309 = global read "G_rio.vi" "LCM_GGA_T"() -> (w625:T8)
                                n310 = To Long Integer(number=w612) -> (32bit integer=w611:i32)
                                n311 = To Long Integer(number=w610) -> (32bit integer=w609:i32)
                                n312 = To Long Integer(number=w608) -> (32bit integer=w607:i32)
                                n313 = Unbundle By Name(w625) -> ("hash"=w621:i64)
                                n314 = Multiply(x=w600, y=1000000.0) -> (x*y=w598:dbl)
                                n315 = To Quad Integer(1:w598) -> (0:w597:i64)
                                n316 = call "hash.vi"("input"=w621) -> ("output"=w620:i64)  [unwired: 10 in]
                                n317 = local read "map"() -> (w602:i32)
                                n318 = Bundle(cluster=w625, "hash"=w620, "sys time"=w597, "time"=w626, "x"=w615, "y"=w614, "h"=w613, "numSV"=w611, "postype"=w609, "lag"=w607, "hordev"=w606, "lat"=w605, "lon"=w604, "hgt"=w603, "map_idx"=w602) -> (w622:T8)
                                n319 = Flatten To String(anything=w622, prepend array or string size? (T)=FALSE) -> (data string=w618:string)  [unwired: 2 in, 2 out]
                                n320 = global read "G_rio.vi" "LCM"() -> (w617:T4)
                                n321 = call "LCM_send.vi"("DATA"=w618, "ID"="GGA_DGPS", "LCM"=w617) -> ()  [unwired: 6 in, 3 out]
                                }
                                }
                                }
                                }
                                n322 = global write "G_rio.vi" "dgps_pos"(w588) -> ()
                                }
                                frame 99 {
                                n323 = call "novatel_bestvel.vi"("gps_data"=w628) -> ("vel"=w627:dbl[])  [unwired: 10 in]
                                n324 = flat-sequence {
                                tunnel: w627 -> [w630]
                                frame #0 {
                                n325 = Index Array(array=w630, index=1) -> (element=w633:dbl)
                                n326 = Not Equal To 0?(x=w633) -> (x != 0?=w634:bool)
                                n327 = local read "LCM"() -> (w632:bool)
                                n328 = And(x=w634, y=w632) -> (x .and. y?=w629:bool)
                                n329 = case shown="True" w629 {
                                tunnel: w630 -> [_ w653]
                                frame False {
                                }
                                frame True {
                                n330 = Array To Cluster(array=w653) -> (cluster=w652:T9)
                                n331 = Get Date/Time In Seconds() -> (seconds since 1Jan1904=w639:timestamp)
                                n332 = To Double Precision Float(number=w639) -> (double precision float=w638:dbl)
                                n333 = Unbundle(w652) -> ("vel[0]"=w644:dbl, "vel[2]"=w643:dbl, "vel[4]"=w642:dbl, "vel[5]"=w641:dbl, "vel[6]"=w640:dbl)  [unwired: 2 out]
                                n334 = global read "G_rio.vi" "LCM_RMC_T"() -> (w654:T10)
                                n335 = Unbundle By Name(w654) -> ("hash"=w650:i64)
                                n336 = Multiply(x=w638, y=1000000.0) -> (x*y=w636:dbl)
                                n337 = call "hash.vi"("input"=w650) -> ("output"=w649:i64)  [unwired: 10 in]
                                n338 = To Quad Integer(1:w636) -> (0:w635:i64)
                                n339 = Bundle(cluster=w654, "hash"=w649, "sys time"=w635, "time"=w644, "speed"=w643, "heading"=w642, "lat"=w641, "lon"=w640) -> (w645:T10)
                                n340 = Flatten To String(anything=w645, prepend array or string size? (T)=FALSE) -> (data string=w647:string)  [unwired: 2 in, 2 out]
                                n341 = global read "G_rio.vi" "LCM"() -> (w646:T4)
                                n342 = call "LCM_send.vi"("DATA"=w647, "ID"="RMC_1", "LCM"=w646) -> ()  [unwired: 6 in, 3 out]
                                }
                                }
                                }
                                }
                                n343 = global write "G_rio.vi" "dgps_vel"(w627) -> ()
                                }
                                }
                                }
                                frame True {
                                }
                                }
                              }
                            }
                          }
                        }
                      }
                      frame True {
                        n344 = xnode "Invoke Method"("FPGA VI Reference In"=w655, "Number of Elements"=u32 1, "Timeout (ms)"=5) -> ("FPGA VI Reference Out"=w659:refnum<k20>, "error out"=w660:errorcluster, "Elements Remaining"=w661:u32)  [unwired: 1 in, 1 out]
                        n345 = xnode "Invoke Method"("FPGA VI Reference In"=w659, "error in"=w660, "Number of Elements"=w661, "Timeout (ms)"=5) -> ()  [unwired: 4 out]
                      }
                    }
                  }
                }
              }
            }
            frame Disabled {
              n346 = while {
                stop <- FALSE stop-if-true
                n347 = flat-sequence {
                  frame #0 {
                    n348 = Wait Until Next ms Multiple(millisecond multiple=u32 100) -> (millisecond timer value=w663:u32)
                    n349 = flat-sequence {
                      tunnel: w663 -> [w666]
                      frame #0 {
                        n350 = feedback #3(w666) -> (w667:u32)
                        n351 = feedback-in #3(w666) -> ()
                        n352 = Subtract(x=w666, y=w667) -> (x-y=→"GPS_novatel_time":u32)
                      }
                    }
                  }
                  frame #1 {
                    n353 = local read "FPGA VI Reference Out"() -> (w670:refnum<k20>)
                    n354 = xnode "Read/Write Control"("FPGA VI Reference In"=w670) -> ("FPGA VI Reference Out"=w669:refnum<k20>, "error out"=w668:errorcluster)  [unwired: 1 in, 1 out]
                    n355 = flat-sequence {
                      tunnel: w669 -> [w681]
                      tunnel: w668 -> [w680]
                      frame #0 {
                        n356 = xnode "Invoke Method"("FPGA VI Reference In"=w681, "error in"=w680, "Number of Elements"=u32 0, "Timeout (ms)"=10) -> ("FPGA VI Reference Out"=w679:refnum<k20>, "error out"=w678:errorcluster, "Elements Remaining"=w677:u32)  [unwired: 1 out]
                        n357 = xnode "Invoke Method"("FPGA VI Reference In"=w679, "error in"=w678, "Number of Elements"=w677) -> ("Data"=w671:u8[])  [unwired: 1 in, 3 out]
                        n358 = local read "rest"() -> (w673:u8[])
                        n359 = Build Array (concatenate)(w673, w671) -> (w672:u8[])
                        n360 = Empty Array?(array=w672) -> (empty?=w674:bool)
                        n361 = case shown="False" w674 {
                          tunnel: w672 -> [w684 _]
                          frame False {
                            n362 = for {
                              N: 2 -> [_]
                              shift-right: [w688] -> w682
                              shift-left: w684 -> [w686]
                              n363 = for {
                                tunnel: w686 -> [w799]
                                tunnel: u8[] [170, 68, 18, 28] -> [w797] mode=indexing
                                shift-right: [w796] -> _
                                shift-left: 0 ("start index (0)") -> [w798]
                                tunnel: [w796] -> w695 mode=indexing
                                n364 = Search 1D Array(1D array=w799, element=w797, start index (0)=w798) -> (index of element=w796:i32)
                              }
                              n365 = Index Array(array=w695, index #1=3 ("index"), index #2=0 ("index")) -> (element #1=w692:i32, element #2=w685:i32)
                              n366 = Subtract(x=w692, y=w685) -> (x-y=w691:i32)
                              n367 = Array Subset(array=w686, index=w685) -> (w687:u8[])  [unwired: 1 in]
                              n368 = Equal?(x=3, y=w691) -> (x = y?=w689:bool)
                              n369 = case shown="True" w689 {
                                tunnel: w687 -> [w701 w710]
                                tunnel: [w700 w707] -> w688
                                tunnel: w685 -> [w699 _]
                                frame False {
                                n370 = Greater Or Equal To 0?(x=w699) -> (x >= 0?=w698:bool)
                                n371 = case shown="False" w698 {
                                tunnel: w701 -> [w702 w705]
                                tunnel: [w702 w703] -> w700
                                frame False {
                                }
                                frame True {
                                n372 = Array Subset(array=w705, index=1 ("length")) -> (w703:u8[])  [unwired: 1 in]
                                }
                                }
                                }
                                frame True {
                                w706 = 4 ("index")
                                n373 = Array Size(array=w710) -> (size(s)=w712:i32)
                                n374 = Increment(x=w706) -> (x+1=w722:i32)
                                n375 = Add(x=w706, y=4) -> (x+y=w719:i32)
                                n376 = Increment(x=w719) -> (x+1=w720:i32)
                                n377 = Index Array(array=w710, index #1=w722, index #2=w706, index #3=w720, index #4=w719) -> (element #1=w718:u8, element #2=w717:u8, element #3=w716:u8, element #4=w715:u8)
                                n378 = Join Numbers(hi=w718, lo=w717) -> ((hi.lo)=w708:u16)
                                n379 = Join Numbers(hi=w716, lo=w715) -> ((hi.lo)=w714:u16)
                                n380 = Add(x=w714, y=u16 32) -> (x+y=w709:u16)
                                n381 = Greater Or Equal?(x=w712, y=w709) -> (x >= y?=w711:bool)
                                n382 = case shown="True" w711 {
                                tunnel: w710 -> [_ w728]
                                tunnel: w709 -> [_ w727]
                                tunnel: w708 -> [_ w724]
                                tunnel: [_ w723] -> w707
                                frame False {
                                }
                                frame True {
                                n383 = Delete From Array(array=w728, length=w727, index=0) -> (deleted portion=w725:u8[], array with subset deleted=w723:u8[])
                                n384 = case shown="99" w724 {
                                tunnel: w725 -> [_ w731 w769]
                                frame 0, Default {
                                }
                                frame 42 {
                                n385 = local read "ecef ref"() -> (w730:dbl[])
                                n386 = call "novatel_bestpos.vi"("ecef ref"=w730, "gps_data"=w731) -> ("LCC"=w729:dbl[])  [unwired: 9 in]
                                n387 = flat-sequence {
                                tunnel: w729 -> [w734]
                                frame #0 {
                                n388 = Index Array(array=w734, index=1) -> (element=w737:dbl)
                                n389 = Not Equal To 0?(x=w737) -> (x != 0?=w733:bool)
                                n390 = local read "LCM"() -> (w736:bool)
                                n391 = And(x=w733, y=w736) -> (x .and. y?=w732:bool)
                                n392 = case shown="True" w732 {
                                tunnel: w734 -> [_ w757]
                                frame False {
                                }
                                frame True {
                                n393 = Array To Cluster(array=w757) -> (cluster=w765:T7)
                                n394 = Get Date/Time In Seconds() -> (seconds since 1Jan1904=w742:timestamp)
                                n395 = To Double Precision Float(number=w742) -> (double precision float=w741:dbl)
                                n396 = Unbundle(w765) -> ("LCC[0]"=w767:dbl, "LCC[2]"=w756:dbl, "LCC[3]"=w755:dbl, "LCC[4]"=w754:dbl, "LCC[6]"=w753:dbl, "LCC[7]"=w751:dbl, "LCC[8]"=w749:dbl, "LCC[9]"=w747:dbl, "LCC[12]"=w746:dbl, "LCC[13]"=w745:dbl, "LCC[14]"=w744:dbl)  [unwired: 4 out]
                                n397 = global read "G_rio.vi" "LCM_GGA_T"() -> (w766:T8)
                                n398 = To Long Integer(number=w753) -> (32bit integer=w752:i32)
                                n399 = To Long Integer(number=w751) -> (32bit integer=w750:i32)
                                n400 = To Long Integer(number=w749) -> (32bit integer=w748:i32)
                                n401 = Unbundle By Name(w766) -> ("hash"=w762:i64)
                                n402 = Multiply(x=w741, y=1000000.0) -> (x*y=w739:dbl)
                                n403 = To Quad Integer(1:w739) -> (0:w738:i64)
                                n404 = call "hash.vi"("input"=w762) -> ("output"=w761:i64)  [unwired: 10 in]
                                n405 = local read "map"() -> (w743:i32)
                                n406 = Bundle(cluster=w766, "hash"=w761, "sys time"=w738, "time"=w767, "x"=w756, "y"=w755, "h"=w754, "numSV"=w752, "postype"=w750, "lag"=w748, "hordev"=w747, "lat"=w746, "lon"=w745, "hgt"=w744, "map_idx"=w743) -> (w763:T8)
                                n407 = Flatten To String(anything=w763, prepend array or string size? (T)=FALSE) -> (data string=w759:string)  [unwired: 2 in, 2 out]
                                n408 = global read "G_rio.vi" "LCM"() -> (w758:T4)
                                n409 = call "LCM_send.vi"("DATA"=w759, "ID"="GGA_DGPS", "LCM"=w758) -> ()  [unwired: 6 in, 3 out]
                                }
                                }
                                }
                                }
                                n410 = global write "G_rio.vi" "dgps_pos"(w729) -> ()
                                }
                                frame 99 {
                                n411 = call "novatel_bestvel.vi"("gps_data"=w769) -> ("vel"=w768:dbl[])  [unwired: 10 in]
                                n412 = flat-sequence {
                                tunnel: w768 -> [w772]
                                frame #0 {
                                n413 = Index Array(array=w772, index=1) -> (element=w774:dbl)
                                n414 = Not Equal To 0?(x=w774) -> (x != 0?=w775:bool)
                                n415 = local read "LCM"() -> (w770:bool)
                                n416 = And(x=w775, y=w770) -> (x .and. y?=w771:bool)
                                n417 = case shown="True" w771 {
                                tunnel: w772 -> [_ w794]
                                frame False {
                                }
                                frame True {
                                n418 = Array To Cluster(array=w794) -> (cluster=w793:T9)
                                n419 = Get Date/Time In Seconds() -> (seconds since 1Jan1904=w780:timestamp)
                                n420 = To Double Precision Float(number=w780) -> (double precision float=w779:dbl)
                                n421 = Unbundle(w793) -> ("vel[0]"=w785:dbl, "vel[2]"=w784:dbl, "vel[4]"=w783:dbl, "vel[5]"=w782:dbl, "vel[6]"=w781:dbl)  [unwired: 2 out]
                                n422 = global read "G_rio.vi" "LCM_RMC_T"() -> (w795:T10)
                                n423 = Unbundle By Name(w795) -> ("hash"=w791:i64)
                                n424 = Multiply(x=w779, y=1000000.0) -> (x*y=w777:dbl)
                                n425 = To Quad Integer(1:w777) -> (0:w776:i64)
                                n426 = call "hash.vi"("input"=w791) -> ("output"=w790:i64)  [unwired: 10 in]
                                n427 = Bundle(cluster=w795, "hash"=w790, "sys time"=w776, "time"=w785, "speed"=w784, "heading"=w783, "lat"=w782, "lon"=w781) -> (w786:T10)
                                n428 = Flatten To String(anything=w786, prepend array or string size? (T)=FALSE) -> (data string=w788:string)  [unwired: 2 in, 2 out]
                                n429 = global read "G_rio.vi" "LCM"() -> (w787:T4)
                                n430 = call "LCM_send.vi"("DATA"=w788, "ID"="RMC_DGPS", "LCM"=w787) -> ()  [unwired: 6 in, 3 out]
                                }
                                }
                                }
                                }
                                n431 = global write "G_rio.vi" "dgps_vel"(w768) -> ()
                                }
                                }
                                }
                                }
                                }
                              }
                            }
                            "rest" <- w682
                          }
                          frame True {
                          }
                        }
                      }
                    }
                  }
                }
              }
            }
            frame Enabled {
            }
          }
          n432 = disable-structure shown="Enabled" {
            frame Enabled {
              n433 = while {
                stop <- FALSE stop-if-true
                n434 = flat-sequence {
                  frame #0 {
                    n435 = Wait Until Next ms Multiple(millisecond multiple=u32 50) -> (millisecond timer value=w1247:u32)
                    n436 = flat-sequence {
                      tunnel: w1247 -> [w1250]
                      frame #0 {
                        n437 = feedback #4(w1250) -> (w1251:u32)
                        n438 = feedback-in #4(w1250) -> ()
                        n439 = Subtract(x=w1250, y=w1251) -> (x-y=→"GPS_Ublox_time 100":u32)
                      }
                    }
                  }
                  frame #1 {
                    n440 = for {
                      N: 5 -> [_]
                      stop <- w1326 stop-if-true
                      n441 = local read "gps2"() -> (w1325:refnum<visa-resource-name>)
                      n442 = local read "ecef ref"() -> (w1331:dbl[])
                      n443 = VISA Read(VISA resource name=w1325, byte count=u32 100) -> (read buffer=w1332:string, error out=w1327:errorcluster)  [unwired: 1 in, 2 out]
                      n444 = Unbundle By Name(w1327) -> ("status"=w1326:bool)
                      n445 = call "nmea.vi"("ecef ref"=w1331, "NMEA"=w1332) -> ("output"=w1329:dbl[], "type"=w1330:u32)  [unwired: 8 in]
                      n446 = case shown="1" w1330 {
                        tunnel: w1329 -> [_ w1333 w1374]
                        frame 0, Default {
                        }
                        frame 1 {
                          n447 = global write "G_rio.vi" "gps_pos 2"(w1333) -> ()
                          n448 = Index Array(array=w1333, index=1) -> (element=w1335:dbl)
                          n449 = Not Equal To 0?(x=w1335) -> (x != 0?=w1334:bool)
                          n450 = local read "LCM"() -> (w1336:bool)
                          n451 = And(x=w1334, y=w1336) -> (x .and. y?=w1338:bool)
                          n452 = case shown="True" w1338 {
                            tunnel: w1333 -> [_ w1358]
                            frame False {
                            }
                            frame True {
                              n453 = Array To Cluster(array=w1358) -> (cluster=w1366:T11)
                              n454 = Get Date/Time In Seconds() -> (seconds since 1Jan1904=w1343:timestamp)
                              n455 = To Double Precision Float(number=w1343) -> (double precision float=w1342:dbl)
                              n456 = Unbundle(w1366) -> ("output[0]"=w1368:dbl, "output[2]"=w1357:dbl, "output[3]"=w1356:dbl, "output[4]"=w1355:dbl, "output[6]"=w1354:dbl, "output[7]"=w1352:dbl, "output[8]"=w1350:dbl, "output[9]"=w1348:dbl, "output[12]"=w1347:dbl, "output[13]"=w1346:dbl, "output[14]"=w1345:dbl)  [unwired: 4 out]
                              n457 = global read "G_rio.vi" "LCM_GGA_T"() -> (w1367:T8)
                              n458 = To Long Integer(number=w1354) -> (32bit integer=w1353:i32)
                              n459 = To Long Integer(number=w1352) -> (32bit integer=w1351:i32)
                              n460 = To Long Integer(number=w1350) -> (32bit integer=w1349:i32)
                              n461 = Unbundle By Name(w1367) -> ("hash"=w1363:i64)
                              n462 = Multiply(x=w1342, y=1000000.0) -> (x*y=w1340:dbl)
                              n463 = call "hash.vi"("input"=w1363) -> ("output"=w1362:i64)  [unwired: 10 in]
                              n464 = To Quad Integer(1:w1340) -> (0:w1339:i64)
                              n465 = local read "map"() -> (w1344:i32)
                              n466 = Bundle(cluster=w1367, "hash"=w1362, "sys time"=w1339, "time"=w1368, "x"=w1357, "y"=w1356, "h"=w1355, "numSV"=w1353, "postype"=w1351, "lag"=w1349, "hordev"=w1348, "lat"=w1347, "lon"=w1346, "hgt"=w1345, "map_idx"=w1344) -> (w1364:T8)
                              n467 = Flatten To String(anything=w1364, prepend array or string size? (T)=FALSE) -> (data string=w1360:string)  [unwired: 2 in, 2 out]
                              n468 = global read "G_rio.vi" "LCM"() -> (w1359:T4)
                              n469 = call "LCM_send.vi"("DATA"=w1360, "ID"="GGA_2", "LCM"=w1359) -> ()  [unwired: 6 in, 3 out]
                            }
                          }
                        }
                        frame 2 {
                          n470 = global write "G_rio.vi" "gps_vel 2"(w1374) -> ()
                          n471 = Index Array(array=w1374, index=1) -> (element=w1371:dbl)
                          n472 = Not Equal To 0?(x=w1371) -> (x != 0?=w1370:bool)
                          n473 = local read "LCM"() -> (w1372:bool)
                          n474 = And(x=w1370, y=w1372) -> (x .and. y?=w1369:bool)
                          n475 = case shown="True" w1369 {
                            tunnel: w1374 -> [_ w1385]
                            frame False {
                            }
                            frame True {
                              n476 = Array To Cluster(array=w1385) -> (cluster=w1387:T12)
                              n477 = Get Date/Time In Seconds() -> (seconds since 1Jan1904=w1379:timestamp)
                              n478 = To Double Precision Float(number=w1379) -> (double precision float=w1378:dbl)
                              n479 = Unbundle(w1387) -> ("output[0]"=w1384:dbl, "output[2]"=w1383:dbl, "output[4]"=w1382:dbl, "output[5]"=w1381:dbl, "output[6]"=w1380:dbl)  [unwired: 2 out]
                              n480 = global read "G_rio.vi" "LCM_RMC_T"() -> (w1386:T10)
                              n481 = Unbundle By Name(w1386) -> ("hash"=w1390:i64)
                              n482 = Multiply(x=w1378, y=1000000.0) -> (x*y=w1376:dbl)
                              n483 = call "hash.vi"("input"=w1390) -> ("output"=w1391:i64)  [unwired: 10 in]
                              n484 = To Quad Integer(1:w1376) -> (0:w1375:i64)
                              n485 = Bundle(cluster=w1386, "hash"=w1391, "sys time"=w1375, "time"=w1384, "speed"=w1383, "heading"=w1382, "lat"=w1381, "lon"=w1380) -> (w1389:T10)
                              n486 = Flatten To String(anything=w1389, prepend array or string size? (T)=FALSE) -> (data string=w1393:string)  [unwired: 2 in, 2 out]
                              n487 = global read "G_rio.vi" "LCM"() -> (w1394:T4)
                              n488 = call "LCM_send.vi"("DATA"=w1393, "ID"="RMC_2", "LCM"=w1394) -> ()  [unwired: 6 in, 3 out]
                            }
                          }
                        }
                      }
                    }
                    n489 = for {
                      N: 5 -> [_]
                      stop <- w1255 stop-if-true
                      n490 = local read "gps1"() -> (w1254:refnum<visa-resource-name>)
                      n491 = local read "ecef ref"() -> (w1259:dbl[])
                      n492 = VISA Read(VISA resource name=w1254, byte count=u32 100) -> (read buffer=w1258:string, error out=w1256:errorcluster)  [unwired: 1 in, 2 out]
                      n493 = Unbundle By Name(w1256) -> ("status"=w1255:bool)
                      n494 = call "nmea.vi"("ecef ref"=w1259, "NMEA"=w1258) -> ("output"=w1261:dbl[], "type"=w1260:u32)  [unwired: 8 in]
                      n495 = case shown="2" w1260 {
                        tunnel: w1261 -> [_ w1263 w1298]
                        frame 0, Default {
                        }
                        frame 1 {
                          n496 = global write "G_rio.vi" "gps_pos 1"(w1263) -> ()
                          n497 = Index Array(array=w1263, index=1) -> (element=w1266:dbl)
                          n498 = Not Equal To 0?(x=w1266) -> (x != 0?=w1267:bool)
                          n499 = local read "LCM"() -> (w1265:bool)
                          n500 = And(x=w1267, y=w1265) -> (x .and. y?=w1262:bool)
                          n501 = case shown="True" w1262 {
                            tunnel: w1263 -> [_ w1287]
                            frame False {
                            }
                            frame True {
                              n502 = Array To Cluster(array=w1287) -> (cluster=w1295:T11)
                              n503 = Get Date/Time In Seconds() -> (seconds since 1Jan1904=w1272:timestamp)
                              n504 = To Double Precision Float(number=w1272) -> (double precision float=w1271:dbl)
                              n505 = Unbundle(w1295) -> ("output[0]"=w1297:dbl, "output[2]"=w1286:dbl, "output[3]"=w1285:dbl, "output[4]"=w1284:dbl, "output[6]"=w1283:dbl, "output[7]"=w1281:dbl, "output[8]"=w1279:dbl, "output[9]"=w1277:dbl, "output[12]"=w1276:dbl, "output[13]"=w1275:dbl, "output[14]"=w1274:dbl)  [unwired: 4 out]
                              n506 = global read "G_rio.vi" "LCM_GGA_T"() -> (w1296:T8)
                              n507 = To Long Integer(number=w1283) -> (32bit integer=w1282:i32)
                              n508 = To Long Integer(number=w1281) -> (32bit integer=w1280:i32)
                              n509 = To Long Integer(number=w1279) -> (32bit integer=w1278:i32)
                              n510 = Unbundle By Name(w1296) -> ("hash"=w1292:i64)
                              n511 = Multiply(x=w1271, y=1000000.0) -> (x*y=w1269:dbl)
                              n512 = call "hash.vi"("input"=w1292) -> ("output"=w1291:i64)  [unwired: 10 in]
                              n513 = To Quad Integer(1:w1269) -> (0:w1268:i64)
                              n514 = local read "map"() -> (w1273:i32)
                              n515 = Bundle(cluster=w1296, "hash"=w1291, "sys time"=w1268, "time"=w1297, "x"=w1286, "y"=w1285, "h"=w1284, "numSV"=w1282, "postype"=w1280, "lag"=w1278, "hordev"=w1277, "lat"=w1276, "lon"=w1275, "hgt"=w1274, "map_idx"=w1273) -> (w1293:T8)
                              n516 = Flatten To String(anything=w1293, prepend array or string size? (T)=FALSE) -> (data string=w1289:string)  [unwired: 2 in, 2 out]
                              n517 = global read "G_rio.vi" "LCM"() -> (w1288:T4)
                              n518 = call "LCM_send.vi"("DATA"=w1289, "ID"="GGA_1", "LCM"=w1288) -> ()  [unwired: 6 in, 3 out]
                            }
                          }
                        }
                        frame 2 {
                          n519 = flat-sequence {
                            tunnel: w1298 -> [w1300]
                            frame #0 {
                              n520 = Index Array(array=w1300, index=1) -> (element=w1303:dbl)
                              n521 = Not Equal To 0?(x=w1303) -> (x != 0?=w1304:bool)
                              n522 = local read "LCM"() -> (w1302:bool)
                              n523 = And(x=w1304, y=w1302) -> (x .and. y?=w1299:bool)
                              n524 = case shown="True" w1299 {
                                tunnel: w1300 -> [_ w1323]
                                frame False {
                                }
                                frame True {
                                n525 = Array To Cluster(array=w1323) -> (cluster=w1322:T12)
                                n526 = Get Date/Time In Seconds() -> (seconds since 1Jan1904=w1309:timestamp)
                                n527 = To Double Precision Float(number=w1309) -> (double precision float=w1308:dbl)
                                n528 = Unbundle(w1322) -> ("output[0]"=w1314:dbl, "output[2]"=w1313:dbl, "output[4]"=w1312:dbl, "output[5]"=w1311:dbl, "output[6]"=w1310:dbl)  [unwired: 2 out]
                                n529 = global read "G_rio.vi" "LCM_RMC_T"() -> (w1324:T10)
                                n530 = Unbundle By Name(w1324) -> ("hash"=w1320:i64)
                                n531 = Multiply(x=w1308, y=1000000.0) -> (x*y=w1306:dbl)
                                n532 = To Quad Integer(1:w1306) -> (0:w1305:i64)
                                n533 = call "hash.vi"("input"=w1320) -> ("output"=w1319:i64)  [unwired: 10 in]
                                n534 = Bundle(cluster=w1324, "hash"=w1319, "sys time"=w1305, "time"=w1314, "speed"=w1313, "heading"=w1312, "lat"=w1311, "lon"=w1310) -> (w1315:T10)
                                n535 = Flatten To String(anything=w1315, prepend array or string size? (T)=FALSE) -> (data string=w1317:string)  [unwired: 2 in, 2 out]
                                n536 = global read "G_rio.vi" "LCM"() -> (w1316:T4)
                                n537 = call "LCM_send.vi"("DATA"=w1317, "ID"="RMC_1", "LCM"=w1316) -> ()  [unwired: 6 in, 3 out]
                                }
                              }
                            }
                          }
                          n538 = global write "G_rio.vi" "gps_vel 1"(w1298) -> ()
                        }
                      }
                    }
                  }
                }
              }
            }
            frame Disabled {
            }
          }
          n539 = while {
            shift-right: [w804] -> _
            shift-left: dbl[] [0.0, 0.0, 0.0, 0.0, 0.0] ("pos(i)") -> [w803]
            stop <- FALSE stop-if-true
            n540 = flat-sequence {
              tunnel: [w810] -> w800
              tunnel: w803 -> [w810]
              tunnel: w800 -> [w816]
              tunnel: [w817] -> w801
              tunnel: [w1186] -> w804
              tunnel: w801 -> [w1186]
              frame #0 {
                n541 = global read "G_rio.vi" "timestamp"() -> (w808:timestamp)
                n542 = Wait Until Next ms Multiple(millisecond multiple=u32 10) -> (millisecond timer value=w805:u32)
                n543 = feedback-in #5(w808) -> ()
                n544 = feedback #5(w808) -> (w809:timestamp)
                n545 = flat-sequence {
                  tunnel: w805 -> [w813]
                  frame #0 {
                    n546 = feedback #6(w813) -> (w814:u32)
                    n547 = feedback-in #6(w813) -> ()
                    n548 = Subtract(x=w813, y=w814) -> (x-y=w812:u32)
                    n549 = To Long Integer(number=w812) -> (32bit integer=→"Pos_time 10":i32)
                  }
                }
                n550 = Subtract(x=w808, y=w809) -> (x-y=→"dt":dbl)
              }
              frame #1 {
                n551 = flat-sequence {
                  tunnel: w816 -> [w829]
                  tunnel: [w829] -> w815
                  tunnel: [w934] -> w817
                  tunnel: w815 -> [w935]
                  frame #0 {
                    n552 = global read "G_rio.vi" "VS_CAN"() -> (w821:dbl)
                    n553 = case shown="True" "ublox" {
                      tunnel: [w830 w847] -> w825
                      tunnel: [w831 w843] -> w820
                      frame False {
                        n554 = global read "G_rio.vi" "dgps_vel"() -> (w842:dbl[])
                        n555 = Index Array(array=w842, index #1=0 ("index"), index #2=1 ("index"), index #3=4 ("index")) -> (element #1=w833:dbl, element #2=w838:dbl, element #3=w835:dbl)
                        n556 = call "angleconv.vi"("deg"=w835) -> ("rad"=w831:dbl)  [unwired: 9 in, 1 out]
                        n557 = feedback #7(0.0 ("Real Matrix Element")) -> (w832:dbl)
                        n558 = feedback-in #7(w833) -> ()
                        n559 = Not Equal?(x=w833, y=w832) -> (x != y?=w839:bool)
                        n560 = Not Equal To 0?(x=w838) -> (x != 0?=w837:bool)
                        n561 = And(x=w839, y=w837) -> (x .and. y?=w830:bool)
                      }
                      frame True {
                        n562 = global read "G_rio.vi" "gps_vel 1"() -> (w871:dbl[])
                        n563 = global read "G_rio.vi" "gps_vel 2"() -> (w850:dbl[])
                        n564 = Index Array(array=w871, index #1=0 ("index"), index #2=1 ("index"), index #3=4 ("index")) -> (element #1=w862:dbl, element #2=w867:dbl, element #3=w864:dbl)
                        n565 = Index Array(array=w850, index #1=0 ("index"), index #2=1 ("index"), index #3=4 ("index")) -> (element #1=w859:dbl, element #2=w854:dbl, element #3=w857:dbl)
                        n566 = call "angleconv.vi"("deg"=w864) -> ("rad"=w846:dbl)  [unwired: 9 in, 1 out]
                        n567 = call "angleconv.vi"("deg"=w857) -> ("rad"=w845:dbl)  [unwired: 9 in, 1 out]
                        n568 = feedback #8(0.0 ("Real Matrix Element")) -> (w861:dbl)
                        n569 = feedback-in #8(w862) -> ()
                        n570 = feedback #9(0.0 ("Real Matrix Element")) -> (w860:dbl)
                        n571 = feedback-in #9(w859) -> ()
                        n572 = Not Equal?(x=w862, y=w861) -> (x != y?=w868:bool)
                        n573 = Not Equal?(x=w859, y=w860) -> (x != y?=w853:bool)
                        n574 = call "headingweightsum.vi"("a"=0.5, "h1"=w845, "h2"=w846) -> ("a*h2+(1-a)*h1"=w843:dbl)  [unwired: 8 in]
                        n575 = Not Equal To 0?(x=w867) -> (x != 0?=w866:bool)
                        n576 = Not Equal To 0?(x=w854) -> (x != 0?=w855:bool)
                        n577 = And(x=w868, y=w866) -> (x .and. y?=w849:bool)
                        n578 = And(x=w853, y=w855) -> (x .and. y?=w848:bool)
                        n579 = And(x=w849, y=w848) -> (x .and. y?=w847:bool)
                      }
                    }
                    "get heading" <- w825
                    n580 = case shown="True" "ublox" {
                      tunnel: [w873 w906] -> w827
                      tunnel: [w874 w901] -> w826
                      tunnel: [w872 w890] -> _
                      frame False {
                        n581 = global read "G_rio.vi" "dgps_pos"() -> (w874:dbl[])
                        n582 = Index Array(array=w874, index #1=0 ("index"), index #2=1 ("index"), index #3=9 ("index")) -> (element #1=w877:dbl, element #2=w880:dbl, element #3=w883:dbl, element #4=w884:dbl)  [unwired: 1 in]
                        n583 = Square(x=w883) -> (x^2=w885:dbl)
                        n584 = Square(x=w884) -> (x^2=w886:dbl)
                        n585 = feedback #10() -> (w876:dbl)  [unwired: 1 in]
                        n586 = feedback-in #10(w877) -> ()
                        n587 = Not Equal?(x=w877, y=w876) -> (x != y?=w878:bool)
                        n588 = Add(x=w885, y=w886) -> (x+y=w887:dbl)
                        n589 = Not Equal To 0?(x=w880) -> (x != 0?=w881:bool)
                        n590 = And(x=w878, y=w881) -> (x .and. y?=w873:bool)
                        n591 = Square Root(x=w887) -> (sqrt(x)=w872:dbl)
                      }
                      frame True {
                        n592 = global read "G_rio.vi" "gps_pos 1"() -> (w921:dbl[])
                        n593 = global read "G_rio.vi" "gps_pos 2"() -> (w908:dbl[])
                        n594 = Add(x=w921, y=w908) -> (x+y=w923:dbl[])
                        n595 = Index Array(array=w921, index #1=0 ("index"), index #3=9 ("index"), index #4=7 ("index")) -> (element #1=w920:dbl, element #2=w919:dbl, element #3=w903:dbl, element #4=w898:dbl)  [unwired: 1 in]
                        n596 = Index Array(array=w908, index #1=0 ("index"), index #3=9 ("index"), index #4=7 ("index")) -> (element #1=w909:dbl, element #2=w910:dbl, element #3=w902:dbl, element #4=w895:dbl)  [unwired: 1 in]
                        n597 = feedback #11(w920) -> (w918:dbl)
                        n598 = feedback-in #11(w920) -> ()
                        n599 = feedback #12(w909) -> (w911:dbl)
                        n600 = feedback-in #12(w909) -> ()
                        n601 = Max & Min(x=w903, y=w902) -> (max(x,y)=w890:dbl)  [unwired: 1 out]
                        n602 = Greater?(x=w898, y=10.0) -> (0:w894:bool)
                        n603 = Greater?(x=w895, y=10.0) -> (0:w893:bool)
                        n604 = Multiply(x=w923, y=0.5) -> (x*y=w901:dbl[])
                        n605 = Not Equal?(x=w920, y=w918) -> (x != y?=w917:bool)
                        n606 = Not Equal?(x=w909, y=w911) -> (x != y?=w912:bool)
                        n607 = And(x=w894, y=w893) -> (x .and. y?=w892:bool)
                        n608 = Not Equal To 0?(x=w919) -> (x != 0?=w916:bool)
                        n609 = Not Equal To 0?(x=w910) -> (x != 0?=w913:bool)
                        n610 = Less?(x=w890, y=1.0) -> (x < y?=w888:bool)
                        n611 = And(x=w917, y=w916) -> (x .and. y?=w891:bool)
                        n612 = And(x=w912, y=w913) -> (x .and. y?=w907:bool)
                        n613 = disable-structure shown="Enabled" {
                          disable-tunnel: w907 -> [w928 w929]
                          disable-tunnel: [w927 w930] -> w906
                          disable-tunnel: w892 -> [w926 _]
                          disable-tunnel: w891 -> [w925 w931]
                          disable-tunnel: w888 -> [w924 _]
                          frame Disabled {
                            n614 = Compound Arithmetic op=AND(w924, w925, w928, w926) -> (w927:bool)
                          }
                          frame Enabled {
                            n615 = And(x=w931, y=w929) -> (x .and. y?=w930:bool)
                          }
                        }
                      }
                    }
                    "pos_gps" <- w826
                    "get position" <- w827
                    n616 = Greater Or Equal To 0?(x=w821) -> (x >= 0?=w822:bool)
                    n617 = Select(t=0.0, s=w822, f=3.141592653589793) -> (s? t:f=w819:dbl)
                    n618 = call "headingoperater.vi"("h1"=w819, "h2"=w820) -> ("h2-h1"=→"h_gps":dbl)  [unwired: 8 in, 1 out]
                  }
                  frame #1 {
                    n619 = local read "dt"() -> (w933:dbl)
                    n620 = Greater Than 0?(x=w933) -> (x > 0?=w932:bool)
                    n621 = case shown="True" w932 {
                      tunnel: w935 -> [w936 w939]
                      tunnel: [w936 w938] -> w934
                      frame False {
                      }
                      frame True {
                        n622 = flat-sequence {
                          tunnel: w939 -> [w976]
                          tunnel: [w944] -> w937
                          tunnel: [w988] -> w938
                          tunnel: w937 -> [w987]
                          frame #0 {
                            n623 = Index Array(array=w976, index #1=0 ("index"), index #2=3 ("index"), index #3=1 ("index"), index #4=3 ("index")) -> (element #1=w970:dbl, element #2=w968:dbl, element #3=w964:dbl, element #4=w951:dbl)
                            n624 = global read "G_rio.vi" "yaw_rate"() -> (w957:dbl)
                            n625 = global read "G_rio.vi" "VS_CAN"() -> (w978:dbl)
                            n626 = global read "G_rio.vi" "VS_CAN"() -> (w960:dbl)
                            n627 = global read "G_rio.vi" "VS_CAN"() -> (w956:dbl)
                            n628 = Negate(x=w957) -> (-x=w949:dbl)
                            n629 = Not Equal To 0?(x=w956) -> (x != 0?=w955:bool)
                            n630 = Divide(x=w978, y=3.6) -> (x/y=w961:dbl)
                            n631 = Divide(x=w960, y=3.6) -> (x/y=w959:dbl)
                            n632 = local read "dt"() -> (w973:dbl)
                            n633 = Multiply(x=w961, y=w973) -> (x*y=w969:dbl)
                            n634 = Cosine(x=w968) -> (cos(x)=w974:dbl)
                            n635 = call "angleconv.vi"("deg"=w949) -> ("rad"=w952:dbl)  [unwired: 9 in, 1 out]
                            n636 = Sine(x=w968) -> (sin(x)=w967:dbl)
                            n637 = Select(t=w952, s=w955, f=0.0) -> (s? t:f=w947:dbl)
                            n638 = local read "dt"() -> (w948:dbl)
                            n639 = Multiply(x=w974, y=w969) -> (x*y=w971:dbl)
                            n640 = Multiply(x=w969, y=w967) -> (x*y=w966:dbl)
                            n641 = Multiply(x=w948, y=w947) -> (x*y=w941:dbl)
                            "rt" <- w941
                            n642 = Add(x=w970, y=w971) -> (x+y=w963:dbl)
                            n643 = Add(x=w966, y=w964) -> (x+y=w962:dbl)
                            n644 = call "headingoperater.vi"("h1"=w941, "h2"=w951) -> ("h2+h1"=w950:dbl)  [unwired: 8 in, 1 out]
                            n645 = Build Array(w963, w962, w959, w950, w947) -> (w944:dbl[])
                            n646 = Index Array(array=w944, index=3) -> (element=w942:dbl)
                            n647 = local read "h_gps"() -> (w940:dbl)
                            n648 = call "headingoperater.vi"("h1"=w942, "h2"=w940) -> ("h2-h1"=w946:dbl)  [unwired: 8 in, 1 out]
                            n649 = Absolute Value(x=w946) -> (abs(x)=→"kalman heading error":dbl)
                          }
                          frame #1 {
                            n650 = local read "get heading"() -> (w995:bool)
                            n651 = local read "get position"() -> (w994:bool)
                            n652 = local read "Kalman init"() -> (w979:bool)
                            n653 = local read "Kalman init"() -> (w980:bool)
                            n654 = global read "G_rio.vi" "VS_CAN"() -> (w993:dbl)
                            n655 = local read "kalman heading error"() -> (w982:dbl)
                            n656 = case shown="True" w979 {
                              tunnel: w995 -> [w998 w1005]
                              tunnel: w994 -> [w1002 w1004]
                              tunnel: [w996 w1003] -> w990
                              frame False {
                                n657 = local read "kalman heading error"() -> (w999:dbl)
                                n658 = Less?(x=w999, y=0.05) -> (x < y?=w1000:bool)
                                n659 = And(x=w998, y=w1000) -> (x .and. y?=w997:bool)
                                n660 = Or(x=w997, y=w1002) -> (x .or. y?=w996:bool)
                              }
                              frame True {
                                n661 = disable-structure shown="Enabled" {
                                disable-tunnel: w1005 -> [w1008 w1010]
                                disable-tunnel: w1004 -> [w1007 w1009]
                                disable-tunnel: [w1006 w1011] -> w1003
                                frame Disabled {
                                n662 = And(x=w1008, y=w1007) -> (x .and. y?=w1006:bool)
                                }
                                frame Enabled {
                                n663 = Or(x=w1010, y=w1009) -> (x .or. y?=w1011:bool)
                                }
                                }
                              }
                            }
                            n664 = Absolute Value(x=w993) -> (abs(x)=w992:dbl)
                            n665 = Less?(x=w982, y=1.0) -> (x < y?=w981:bool)
                            n666 = Or(x=w981, y=w980) -> (x .or. y?=w984:bool)
                            n667 = Greater?(x=w992, y=5.0) -> (0:w989:bool)
                            n668 = And(x=w990, y=w989) -> (x .and. y?=w985:bool)
                            n669 = And(x=w985, y=w984) -> (x .and. y?=w983:bool)
                            n670 = case shown="True" w983 {
                              tunnel: [w1015 w1041] -> w988
                              tunnel: w987 -> [w1016 w1044]
                              frame False {
                                n671 = local read "Kalman init"() -> (w1018:bool)
                                n672 = global read "G_rio.vi" "VS_CAN"() -> (w1019:dbl)
                                n673 = Equal To 0?(x=w1019) -> (x = 0?=w1017:bool)
                                n674 = And(x=w1018, y=w1017) -> (x .and. y?=w1014:bool)
                                n675 = Or(x=w1014, y="GPS init") -> (x .or. y?=w1013:bool)
                                n676 = case shown="True" w1013 {
                                tunnel: w1016 -> [w1020 w1021]
                                tunnel: [w1020 w1023] -> w1015
                                tunnel: "GPS init" -> [_ w1022]
                                frame False {
                                }
                                frame True {
                                n677 = case shown="False" w1022 {
                                tunnel: [w1034 w1040] -> w1023
                                tunnel: w1021 -> [w1029 _]
                                frame True {
                                n678 = Index Array(array=w1029, index #1=2 ("index")) -> (element #1=w1027:dbl, element #2=w1026:dbl, element #3=w1025:dbl)  [unwired: 2 in]
                                n679 = local write "GPS init"(FALSE ("GPS init")) -> ()
                                n680 = local read "pos_gps"() -> (w1030:dbl[])
                                n681 = Index Array(array=w1030, index #1=2 ("index")) -> (element #1=w1032:dbl, element #2=w1031:dbl)  [unwired: 1 in]
                                n682 = Build Array(w1032, w1031, w1027, w1026, w1025) -> (w1034:dbl[])
                                }
                                frame False {
                                w1036 = 0.0 ("element")
                                n683 = local read "pos_gps"() -> (w1035:dbl[])
                                n684 = Index Array(array=w1035, index #1=2 ("index")) -> (element #1=w1038:dbl, element #2=w1037:dbl)  [unwired: 1 in]
                                n685 = Build Array(w1038, w1037, w1036, w1036, w1036) -> (w1040:dbl[])
                                }
                                }
                                }
                                }
                              }
                              frame True {
                                n686 = flat-sequence {
                                tunnel: w1044 -> [w1045]
                                tunnel: [w1045] -> w1043
                                tunnel: w1043 -> [w1086]
                                tunnel: [w1086] -> w1042
                                tunnel: w1042 -> [w1113]
                                tunnel: [w1117] -> w1041
                                frame #0 {
                                w1054 = 0.0 ("element")
                                w1058 = 0.0 ("element")
                                w1060 = 0.0 ("element")
                                w1062 = 0.0 ("element")
                                w1064 = 0.0 ("element")
                                n687 = Index Array(array=w1045, index #1=3 ("index"), index #2=2 ("index"), index #3=3 ("index"), index #4=2 ("index")) -> (element #1=w1074:dbl, element #2=w1076:dbl, element #3=w1079:dbl, element #4=w1068:dbl)
                                n688 = Negate(x=w1076) -> (-x=w1075:dbl)
                                n689 = Sine & Cosine(0:w1079) -> (1:w1071:dbl, 2:w1069:dbl)
                                n690 = Multiply(x=w1075, y=w1071) -> (x*y=w1072:dbl)
                                n691 = Multiply(x=w1069, y=w1068) -> (x*y=w1067:dbl)
                                n692 = Cosine(x=w1074) -> (cos(x)=w1073:dbl)
                                n693 = Build Array(w1064, w1064, w1073, w1072, 0.0 ("element")) -> (w1066:dbl[])
                                n694 = Build Array(w1062, w1062, w1071, w1067, 0.0 ("element")) -> (w1065:dbl[])
                                n695 = Build Array(w1060, w1060, w1060, w1060, w1060) -> (w1059:dbl[])
                                n696 = Build Array(w1058, w1058, w1058, w1058, 1.0 ("element")) -> (w1056:dbl[])
                                n697 = Build Array(w1054, w1054, w1054, w1054, w1054) -> (w1055:dbl[])
                                n698 = Build Array(w1066, w1065, w1059, w1056, w1055) -> (w1052:dbl[][])
                                n699 = call-poly <vilib>:"Array To Matrix.vi"("Real 2D Array"=w1052) -> ("Real Matrix"=w1050:T13)
                                n700 = global read "G_rio.vi" "P"() -> (w1053:T13)
                                n701 = Transpose Matrix(1:w1050) -> (0:w1049:T13)
                                n702 = call-poly <vilib>:"Multiply.vi"("Real Matrix B"=w1053, "Real Matrix A"=w1050) -> ("A * B"=w1051:T13)
                                n703 = call-poly <vilib>:"Multiply.vi"("Real Matrix B"=w1049, "Real Matrix A"=w1051) -> ("A * B"=w1048:T13)
                                n704 = global read "G_rio.vi" "Q"() -> (w1047:T13)
                                n705 = call-poly <vilib>:"Add.vi"("Real Matrix B"=w1047, "Real Matrix A"=w1048) -> ("A + B"=w1046:T13)
                                n706 = global write "G_rio.vi" "Pp"(w1046) -> ()
                                }
                                frame #1 {
                                n707 = global read "G_rio.vi" "Pp"() -> (w1111:T13)
                                n708 = global read "G_rio.vi" "H"() -> (w1110:T13)
                                n709 = Array Subset(array=w1086, index=0, length=2) -> (w1093:dbl[])
                                n710 = global read "G_rio.vi" "H"() -> (w1105:T13)
                                n711 = local read "pos_gps"() -> (w1089:dbl[])
                                n712 = global read "G_rio.vi" "Pp"() -> (w1104:T13)
                                n713 = call-poly <vilib>:"Multiply.vi"("Real Matrix B"=w1111, "Real Matrix A"=w1110) -> ("A * B"=w1109:T13)
                                n714 = Transpose Matrix(1:w1110) -> (0:w1108:T13)
                                n715 = Transpose Matrix(1:w1105) -> (0:w1103:T13)
                                n716 = local read "kalman heading error"() -> (w1098:dbl)
                                n717 = call-poly <vilib>:"Multiply.vi"("Real Matrix B"=w1103, "Real Matrix A"=w1104) -> ("A * B"=w1102:T13)
                                n718 = call-poly <vilib>:"Multiply.vi"("Real Matrix B"=w1108, "Real Matrix A"=w1109) -> ("A * B"=w1107:T13)
                                n719 = Array Subset(array=w1089, index=2, length=2) -> (w1092:dbl[])
                                n720 = global read "G_rio.vi" "R"() -> (w1106:T13)
                                n721 = Subtract(x=w1092, y=w1093) -> (x-y=w1094:dbl[])
                                n722 = call-poly <vilib>:"Add.vi"("Real Matrix B"=w1106, "Real Matrix A"=w1107) -> ("A + B"=w1101:T13)
                                n723 = Square(x=w1094) -> (x^2=w1095:dbl[])
                                n724 = Less?(x=w1098, y=0.05) -> (x < y?=w1083:bool)
                                n725 = Add Array Elements(numeric array=w1095) -> (sum=w1096:dbl)
                                n726 = call-poly <vilib>:"Inverse Matrix.vi"("Input Matrix"=w1101) -> ("Inverse Matrix"=w1100:T13)  [unwired: 1 in, 1 out]
                                n727 = call-poly <vilib>:"Multiply.vi"("Real Matrix B"=w1100, "Real Matrix A"=w1102) -> ("A * B"=w1099:T13)
                                n728 = Square Root(x=w1096) -> (sqrt(x)=w1085:dbl)
                                n729 = global write "G_rio.vi" "K"(w1099) -> ()
                                n730 = Less?(x=w1085, y=2.5) -> (x < y?=w1082:bool)
                                n731 = And(x=w1083, y=w1082) -> (x .and. y?=w1081:bool)
                                n732 = case shown="True" w1081 {
                                frame False {
                                }
                                frame True {
                                n733 = local write "Kalman init"(FALSE ("Kalman init")) -> ()
                                }
                                }
                                }
                                frame #2 {
                                n734 = disable-structure shown="Enabled" {
                                disable-tunnel: [w1135 w1136] -> w1115
                                disable-tunnel: w1113 -> [_ w1146]
                                frame Disabled {
                                n735 = local read "get position"() -> (w1135:bool)
                                }
                                frame Enabled {
                                n736 = disable-structure shown="Enabled" {
                                disable-tunnel: [w1152 TRUE ("Kalman init")] -> w1138
                                frame Disabled {
                                n737 = local read "Kalman init"() -> (w1152:bool)
                                }
                                frame Enabled {
                                }
                                }
                                n738 = Array Subset(array=w1146, index=0, length=2) -> (w1144:dbl[])
                                n739 = local read "pos_gps"() -> (w1149:dbl[])
                                n740 = Array Subset(array=w1149, index=2, length=2) -> (w1145:dbl[])
                                n741 = Subtract(x=w1145, y=w1144) -> (x-y=w1143:dbl[])
                                n742 = Square(x=w1143) -> (x^2=w1142:dbl[])
                                n743 = Add Array Elements(numeric array=w1142) -> (sum=w1141:dbl)
                                n744 = Square Root(x=w1141) -> (sqrt(x)=w1140:dbl)
                                "gps pos error" <- w1140
                                n745 = Less?(x=w1140, y=3.0) -> (x < y?=w1137:bool)
                                n746 = Or(x=w1138, y=w1137) -> (x .or. y?=w1136:bool)
                                }
                                }
                                n747 = disable-structure shown="Enabled" {
                                disable-tunnel: [w1129 w1130] -> w1116
                                frame Disabled {
                                n748 = local read "get heading"() -> (w1129:bool)
                                }
                                frame Enabled {
                                n749 = local read "Kalman init"() -> (w1131:bool)
                                n750 = local read "kalman heading error"() -> (w1133:dbl)
                                n751 = Less?(x=w1133, y=0.1) -> (x < y?=w1132:bool)
                                n752 = Or(x=w1132, y=w1131) -> (x .or. y?=w1130:bool)
                                }
                                }
                                n753 = Index Array(array=w1113, index=3) -> (element=w1120:dbl)
                                n754 = global read "G_rio.vi" "K"() -> (w1128:T13)
                                n755 = global read "G_rio.vi" "H"() -> (w1127:T13)
                                n756 = global read "G_rio.vi" "Pp"() -> (w1125:T13)
                                n757 = call-poly <vilib>:"Multiply.vi"("Real Matrix B"=w1127, "Real Matrix A"=w1128) -> ("A * B"=w1126:T13)
                                n758 = call-poly <vilib>:"Multiply.vi"("Real Matrix B"=w1125, "Real Matrix A"=w1126) -> ("A * B"=w1124:T13)
                                n759 = global read "G_rio.vi" "Pp"() -> (w1123:T13)
                                n760 = call-poly <vilib>:"Subtract.vi"("Real Matrix B"=w1124, "Real Matrix A"=w1123) -> ("A - B"=w1122:T13)
                                n761 = global write "G_rio.vi" "P"(w1122) -> ()
                                n762 = case shown="True" w1116 {
                                tunnel: w1120 -> [w1178 w1185]
                                tunnel: [w1178 w1180] -> w1114
                                frame False {
                                }
                                frame True {
                                n763 = global read "G_rio.vi" "K"() -> (w1184:T13)
                                n764 = Index Array(array=w1184, index (row)=3, index (col)=2 ("disabled index (col)")) -> (element=w1181:dbl)
                                n765 = local read "h_gps"() -> (w1179:dbl)
                                n766 = call "headingweightsum2.vi"("a"=w1181, "h2"=w1179, "h1"=w1185) -> ("a*h2+(1-a)*h1"=w1180:dbl)  [unwired: 8 in]
                                }
                                }
                                n767 = case shown="True" w1115 {
                                tunnel: w1113 -> [w1154 w1166]
                                tunnel: [w1154 w1165] -> w1119
                                tunnel: w1114 -> [_ w1155]
                                frame False {
                                }
                                frame True {
                                n768 = disable-structure shown="Enabled" {
                                disable-tunnel: [w1176 w1177] -> w1156
                                disable-tunnel: w1155 -> [_ w1177]
                                frame Disabled {
                                n769 = local read "h_gps"() -> (w1176:dbl)
                                }
                                frame Enabled {
                                }
                                }
                                n770 = call-poly <vilib>:"Array To Matrix.vi"("Real 1D Array"=w1166) -> ("Real Matrix (Column Vector)"=w1170:T13)
                                n771 = local read "pos_gps"() -> (w1160:dbl[])
                                n772 = global read "G_rio.vi" "H"() -> (w1175:T13)
                                n773 = call-poly <vilib>:"Multiply.vi"("Real Matrix B"=w1170, "Real Matrix A"=w1175) -> ("A * B"=w1174:T13)
                                n774 = Array Subset(array=w1160, index=2, length=2) -> (w1161:dbl[])
                                n775 = Build Array (concatenate)(w1161, w1156) -> (w1157:dbl[])
                                n776 = call-poly <vilib>:"Array To Matrix.vi"("Real 1D Array"=w1157) -> ("Real Matrix (Column Vector)"=w1173:T13)
                                n777 = call-poly <vilib>:"Subtract.vi"("Real Matrix B"=w1174, "Real Matrix A"=w1173) -> ("A - B"=w1171:T13)
                                n778 = global read "G_rio.vi" "K"() -> (w1172:T13)
                                n779 = call-poly <vilib>:"Multiply.vi"("Real Matrix B"=w1171, "Real Matrix A"=w1172) -> ("A * B"=w1164:T13)
                                n780 = call-poly <vilib>:"Multiply.vi"("Real Matrix A"=w1164, "Real Scalar c"=0.25) -> ("c * A"=w1162:T13)
                                n781 = call-poly <vilib>:"Add.vi"("Real Matrix B"=w1170, "Real Matrix A"=w1162) -> ("A + B"=w1169:T13)
                                n782 = call-poly <vilib>:"Matrix To Array.vi"("Real Matrix"=w1169) -> ("Real 2D Array"=w1168:dbl[][])
                                n783 = Index Array(array=w1168, index (col)=0 ("disabled index (col)")) -> (element=w1165:dbl[])  [unwired: 1 in]
                                }
                                }
                                n784 = Replace Array Subset(array=w1119, new element=w1114, index=3) -> (w1117:dbl[])
                                }
                                }
                              }
                            }
                          }
                        }
                      }
                    }
                  }
                }
              }
              frame #2 {
                n785 = flat-sequence {
                  tunnel: w1186 -> [w1193]
                  frame #0 {
                    n786 = local read "h_gps"() -> (w1194:dbl)
                    n787 = local read "dt"() -> (w1190:dbl)
                    n788 = Array Subset(array=w1193, index=0, length=2) -> (w1201:dbl[])
                    "pos" <- w1201
                    n789 = Index Array(array=w1193, index=3) -> (element=w1198:dbl)
                    n790 = call "angleconv.vi"("rad"=w1198) -> ("deg"=→"Heading":dbl)  [unwired: 9 in, 1 out]
                    n791 = Greater Than 0?(x=w1190) -> (x > 0?=w1188:bool)
                    n792 = Greater?(x=1.0, y=w1190) -> (0:w1192:bool)
                    n793 = call "headingoperater.vi"("h1"=0.0, "h2"=w1194) -> ("h2+h1"=w1195:dbl)  [unwired: 8 in, 1 out]
                    n794 = local read "LCM"() -> (w1189:bool)
                    n795 = call "angleconv.vi"("rad"=w1195) -> ("deg"=→"H_GPS":dbl)  [unwired: 9 in, 1 out]
                    n796 = Compound Arithmetic op=AND(w1192, w1188, w1189) -> (w1187:bool)
                    n797 = case shown="True" w1187 {
                      tunnel: w1201 -> [w1211 _]
                      tunnel: w1198 -> [w1207 _]
                      tunnel: w1194 -> [w1206 _]
                      tunnel: w1193 -> [_ w1218]
                      frame False {
                        n798 = global read "G_rio.vi" "VS_CAN"() -> (w1204:dbl)
                        n799 = local read "pos_gps"() -> (w1210:dbl[])
                        n800 = Array Subset(array=w1210, index=5, length=10) -> (w1215:dbl[])
                        n801 = Array Subset(array=w1210, index=12, length=3) -> (w1212:dbl[])
                        n802 = local read "map"() -> (w1205:i32)
                        n803 = local read "dt"() -> (w1209:dbl)
                        n804 = Build Array (concatenate)(w1215, w1212, w1211, w1209, w1205, w1204, w1207, w1206) -> (w1208:dbl[])
                        n805 = shared-variable "veloster\\sharedvari.lvlib\\RIONAV"(w1208) -> ()  [unwired: 1 in, 1 out]
                      }
                      frame True {
                        n806 = flat-sequence {
                          tunnel: w1218 -> [w1243]
                          frame #0 {
                            n807 = Array To Cluster(array=w1243) -> (cluster=w1241:T14)
                            n808 = Get Date/Time In Seconds() -> (seconds since 1Jan1904=w1234:timestamp)
                            n809 = local read "Kalman init"() -> (w1223:bool)
                            n810 = local read "file write"() -> (w1224:bool)
                            n811 = To Double Precision Float(number=w1234) -> (double precision float=w1228:dbl)
                            n812 = Unbundle(w1241) -> ("Real 2D Array[0]"=w1233:dbl, "Real 2D Array[1]"=w1232:dbl, "Real 2D Array[2]"=w1231:dbl, "Real 2D Array[3]"=w1230:dbl, "Real 2D Array[4]"=w1229:dbl)
                            n813 = global read "G_rio.vi" "LCM_POS_T"() -> (w1242:T15)
                            n814 = local read "dt"() -> (w1222:dbl)
                            n815 = Select(t=0.0, s=w1223, f=w1222) -> (s? t:f=w1220:dbl)
                            n816 = Unbundle By Name(w1242) -> ("hash"=w1239:i64)
                            n817 = Multiply(x=w1228, y=1000000.0) -> (x*y=w1226:dbl)
                            n818 = To Quad Integer(1:w1226) -> (0:w1225:i64)
                            n819 = call "hash.vi"("input"=w1239) -> ("output"=w1238:i64)  [unwired: 10 in]
                            n820 = Bundle(cluster=w1242, "hash"=w1238, "sys time"=w1225, "dt"=w1220, "x"=w1233, "y"=w1232, "speed"=w1231, "heading"=w1230, "yaw_rate"=w1229) -> (w1219:T15)
                            n821 = case shown="True" w1224 {
                              tunnel: w1219 -> [_ w1244]
                              frame False {
                              }
                              frame True {
                                n822 = local read "data write"() -> (w1245:refnum<file>)
                                n823 = Write to Binary File(file (use dialog)=w1245, data=w1244) -> ()  [unwired: 4 in, 3 out]
                              }
                            }
                            n824 = Flatten To String(anything=w1219, prepend array or string size? (T)=FALSE) -> (data string=w1236:string)  [unwired: 2 in, 2 out]
                            n825 = global read "G_rio.vi" "LCM"() -> (w1235:T4)
                            n826 = call "LCM_send.vi"("DATA"=w1236, "ID"="POS_T", "LCM"=w1235) -> ()  [unwired: 6 in, 3 out]
                          }
                        }
                      }
                    }
                  }
                }
              }
            }
          }
        }
        frame Disabled {
        }
      }
      n827 = while {
        stop <- FALSE stop-if-true
        n828 = flat-sequence {
          frame #0 {
            n829 = Wait Until Next ms Multiple(millisecond multiple=u32 10) -> (millisecond timer value=w155:u32)
            n830 = flat-sequence {
              tunnel: w155 -> [w159]
              frame #0 {
                n831 = feedback #13(w159) -> (w160:u32)
                n832 = feedback-in #13(w159) -> ()
                n833 = Subtract(x=w159, y=w160) -> (x-y=w158:u32)
                n834 = To Long Integer(number=w158) -> (32bit integer=→"Con_time 10":i32)
              }
            }
          }
          frame #1 {
            n835 = flat-sequence {
              frame #0 {
                n836 = local read "LCM"() -> (w180:bool)
                n837 = case shown="True" w180 {
                  frame False {
                    n838 = shared-variable "veloster\\sharedvari.lvlib\\vs_des"() -> (w187:dbl)  [unwired: 1 in, 1 out]
                    n839 = global read "G_rio.vi" "Ref_steer_planner"() -> (w185:dbl)
                    n840 = global read "G_rio.vi" "Ref_vel_planner"() -> (w186:dbl)
                    n841 = shared-variable "veloster\\sharedvari.lvlib\\steer_input"() -> (w184:dbl)  [unwired: 1 in, 1 out]
                    n842 = Not A Number/Path/Refnum?(number/path/refnum=w187) -> (NaN/Path/Refnum?=w188:bool)
                    n843 = Select(t=w186, s=w188, f=w187) -> (s? t:f=w181:dbl)
                    n844 = Not A Number/Path/Refnum?(number/path/refnum=w184) -> (NaN/Path/Refnum?=w183:bool)
                    n845 = global write "G_rio.vi" "Ref_vel_planner"(w181) -> ()
                    n846 = Select(t=w185, s=w183, f=w184) -> (s? t:f=w182:dbl)
                    n847 = global write "G_rio.vi" "Ref_steer_planner"(w182) -> ()
                  }
                  frame True {
                    n848 = global read "G_rio.vi" "LCM PC"() -> (w191:T4)
                    n849 = call "LCM_read.vi"("LCM"=w191) -> ("data"=w189:string, "ID"=w190:string)  [unwired: 7 in, 2 out]
                    n850 = case shown="\"CON_INPUT_T\"" w190 {
                      tunnel: w189 -> [_ w192]
                      frame "False", Default {
                      }
                      frame "CON_INPUT_T" {
                        n851 = global read "G_rio.vi" "CON_INPUT_T"() -> (w194:T16)
                        n852 = Unflatten From String(type=w194, binary string=w192, data includes array or string size? (T)=FALSE) -> (value=w193:T16, error out=w195:errorcluster)  [unwired: 2 in, 1 out]
                        n853 = case shown="No Error" w195 {
                          tunnel: w193 -> [w199 _]
                          frame No Error {
                            n854 = Unbundle By Name(w199) -> ("ref_vel"=w198:dbl, "ref_steer"=w197:dbl)
                            n855 = global write "G_rio.vi" "Ref_vel_planner"(w198) -> ()
                            n856 = global write "G_rio.vi" "Ref_steer_planner"(w197) -> ()
                          }
                          frame Error {
                          }
                        }
                      }
                    }
                  }
                }
              }
            }
            n857 = global read "G_rio.vi" "Throttle_Enable"() -> (→"Throttle Enable":bool)
            n858 = local read "FPGA VI Reference Out"() -> (w177:refnum<k20>)
            n859 = xnode "Read/Write Control"("FPGA VI Reference In"=w177) -> ("Auto"=w162:bool, "Run"=w176:bool, "T Lim"=w178:bool, "brk enc"=w166:u8)  [unwired: 1 in, 2 out]
            "Auto" <- w162
            "brk enc" <- w166
            n860 = global write "G_rio.vi" "Auto"(w162) -> ()
            n861 = global write "G_rio.vi" "T Lim"(w178) -> ()
            n862 = To Double Precision Float(number=w166) -> (double precision float=w174:dbl)
            n863 = And(x=w162, y=w176) -> (x .and. y?=w163:bool)
            "Run" <- w163
            n864 = global write "G_rio.vi" "Run"(w163) -> ()
            n865 = Subtract(x=w174, y=220.0) -> (x-y=w172:dbl)
            n866 = Multiply(x=w172, y=-100.0) -> (x*y=w169:dbl)
            n867 = Not(x=w163) -> (.not. x?=w161:bool)
            n868 = And(x=w162, y=w161) -> (x .and. y?=→"E - STOP":bool)
            n869 = Divide(x=w169, y=175.0) -> (x/y=w168:dbl)
            n870 = In Range and Coerce(upper limit=100.0, x=w168, lower limit=0.0) -> (coerced(x)=w165:dbl)  [unwired: 1 out]
            n871 = global write "G_rio.vi" "brake encoder"(w165) -> ()
          }
          frame #2 {
            n872 = flat-sequence {
              frame #0 {
                n873 = global read "G_rio.vi" "Ref_vel_planner"() -> (w244:dbl)
                n874 = Select(t=w244, s="Velocity input", f="Ref vel manual") -> (s? t:f=w247:dbl)
                n875 = To Long Integer(number=w247) -> (32bit integer=w246:i32)
                n876 = Sign(1:w246) -> (0:w245:i32)
                "P, R, D" <- w245
                n877 = case shown="1" w245 {
                  tunnel: [w251 _ w258] -> w248
                  tunnel: w247 -> [w253 _ w257]
                  frame -1 {
                    n878 = global read "G_rio.vi" "gear selector disp"() -> (w256:u8)
                    n879 = Equal?(x=w256, y=u8 7) -> (x = y?=w254:bool)
                    n880 = Select(t=w253, s=w254, f=0.0) -> (s? t:f=w251:dbl)
                  }
                  frame 0, Default {
                  }
                  frame 1 {
                    n881 = global read "G_rio.vi" "gear selector disp"() -> (w259:u8)
                    n882 = case shown="4, 5" w259 {
                      tunnel: [_ w260] -> w258
                      tunnel: w257 -> [_ w260]
                      frame 0, Default {
                      }
                      frame 4, 5 {
                      }
                    }
                  }
                }
                "Ref vel" <- w248
              }
            }
            n883 = feedback #14(FALSE ("Steer input")) -> (w201:bool)
            n884 = case shown="True" w201 {
              frame False {
              }
              frame True {
                n885 = flat-sequence {
                  frame #0 {
                    n886 = global read "G_rio.vi" "Ref_steer_planner"() -> (w203:dbl)
                    n887 = global read "G_rio.vi" "mdps str_ang"() -> (w209:dbl)
                    n888 = global read "G_rio.vi" "mdps str_ang"() -> (w205:dbl)
                    n889 = Select(t=w203, s="Steer input", f="Ref steer manual") -> (s? t:f=w204:dbl)
                    n890 = Add(x=w209, y=120.0 ("upper limit")) -> (x+y=w213:dbl)
                    n891 = Subtract(x=w205, y=120.0 ("upper limit")) -> (x-y=w211:dbl)
                    n892 = In Range and Coerce(upper limit=w213, x=w204, lower limit=w211) -> (coerced(x)=→"Ref steer":dbl)  [unwired: 1 out]
                  }
                  frame #1 {
                    n893 = local read "Ref steer"() -> (w217:dbl)
                    n894 = feedback #15(u8 0 ("Con steer alivecnt")) -> (w214:u8)
                    n895 = Increment(x=w214) -> (x+1=w215:u8)
                    n896 = feedback-in #15(w215) -> ()
                    n897 = global read "G_rio.vi" "Auto"() -> (w238:bool)
                    n898 = Multiply(x=w217, y=10.0) -> (x*y=w230:dbl)
                    n899 = And(x=w238, y="SPAS Enable") -> (x .and. y?=w240:bool)
                    n900 = Greater Than 0?(x=w230) -> (x > 0?=w231:bool)
                    n901 = Add(x=w230, y=65536.0) -> (x+y=w228:dbl)
                    n902 = Select(t=w230, s=w231, f=w228) -> (s? t:f=w227:dbl)
                    n903 = To Unsigned Word Integer(number=w227) -> (unsigned 16bit integer=w226:u16)
                    n904 = Split Number(x=w226) -> (hi(x)=w225:u8, lo(x)=w224:u8)
                    n905 = Build Array(u8 0 ("Con steer status"), w224, w225, u8 0 ("element"), w214, u8 0 ("element"), u8 0 ("element")) -> (w219:u8[])
                    n906 = Add Array Elements(numeric array=w219) -> (sum=w220:u8)
                    n907 = Build Array (concatenate)(w219, w220) -> (w233:u8[])
                    n908 = Bundle By Name(cluster=T2 {"timestamp"=timestamp(0 s since 1904-01-01), "payload"=[0], "identifier"=912, "type"=0, "extended?"=FALSE, "echo?"=FALSE} ("CAN frame"), "payload"=w233) -> (w235:T2)
                    n909 = Build Array(w235, T2 {"timestamp"=timestamp(0 s since 1904-01-01), "payload"=[0, 0, 0, 0, 0, 0, 0, 0], "identifier"=1285, "type"=0, "extended?"=FALSE, "echo?"=FALSE} ("CAN frame")) -> (w236:T2[])
                    n910 = case shown="True" w240 {
                      tunnel: w236 -> [_ w242]
                      frame False {
                      }
                      frame True {
                        n911 = local read "CAN write"() -> (w241:refnum<k21>)
                        n912 = call-poly <vilib>:"XNET Write.vi"("session in"=w241, "data"=w242, "timeout (10)"=0.01) -> ()  [unwired: 11 in, 2 out]
                      }
                    }
                  }
                }
              }
            }
            n913 = Not(x=w201) -> (.not. x?=w200:bool)
            n914 = feedback-in #14(w200) -> ()
          }
          frame #3 {
            n915 = flat-sequence {
              frame #0 {
                n916 = global read "G_rio.vi" "VS_CAN"() -> (w322:dbl)
                n917 = global read "G_rio.vi" "Brake Encoder mcp"() -> (w321:dbl)
                n918 = global read "G_rio.vi" "brake_act_can"() -> (w320:bool)
                n919 = local read "Ref vel"() -> (w319:dbl)
                n920 = call "B_control.vi"("Ref vel"=w319, "VS_CAN"=w322, "Brake Encoder"=w321, "brake_act_can"=w320) -> ("Ref Brk Enc"=w323:dbl)  [unwired: 15 in]
                n921 = global write "G_rio.vi" "Ref Brk Enc"(w323) -> ()
              }
            }
            n922 = flat-sequence {
              frame #0 {
                n923 = global read "G_rio.vi" "VS_CAN"() -> (w315:dbl)
                n924 = global read "G_rio.vi" "accel pedal value"() -> (w317:dbl)
                n925 = local read "Ref vel"() -> (w314:dbl)
                n926 = call "T_control.vi"("Ref vel"=w314, "VS_CAN"=w315, "accel pedal value"=w317, "pid gain"=dbl[] [3.0, 0.0, 0.3] ("pid gain 1")) -> ("Ref APS"=w318:dbl)  [unwired: 15 in]
                n927 = global write "G_rio.vi" "Ref APS"(w318) -> ()
              }
            }
            n928 = global read "G_rio.vi" "Auto"() -> (w261:bool)
            n929 = case shown="False" w261 {
              tunnel: [w263 w297] -> w262
              frame False {
                n930 = global read "G_rio.vi" "VS_CAN"() -> (w267:dbl)
                n931 = Absolute Value(x=w267) -> (abs(x)=w266:dbl)
                n932 = Less?(x=w266, y=0.05) -> (x < y?=w264:bool)
                n933 = case shown="True" w264 {
                  tunnel: [_ w270] -> w263
                  frame False {
                  }
                  frame True {
                    n934 = Sign(1:"Gear Manual") -> (0:w271:i32)
                    n935 = To Long Integer(number=w271) -> (32bit integer=w269:i32)
                    n936 = case shown="0" w269 {
                      tunnel: [w278 w282 w286] -> w270
                      frame 0 {
                        n937 = global read "G_rio.vi" "gear selector disp"() -> (w276:u8)
                        n938 = Equal To 0?(x=w276) -> (x = 0?=w275:bool)
                        n939 = Equal?(x=u8 7 ("y"), y=w276) -> (x = y?=w280:bool)
                        n940 = Select(t=-1.0, s=w275, f=1.0) -> (s? t:f=w274:dbl)
                        n941 = Select(t=0.0, s=w280, f=w274) -> (s? t:f=w278:dbl)
                      }
                      frame 1, Default {
                        n942 = global read "G_rio.vi" "gear selector disp"() -> (w285:u8)
                        n943 = Equal To 0?(x=w285) -> (x = 0?=w284:bool)
                        n944 = Select(t=0.0, s=w284, f=1.0 ("t")) -> (s? t:f=w282:dbl)
                      }
                      frame -1 {
                        n945 = global read "G_rio.vi" "gear selector disp"() -> (w287:u8)
                        n946 = case shown="3..5, Default" w287 {
                          tunnel: [-1.0 1.0 0.0] -> w286
                          frame 0, 6, 7 {
                          }
                          frame 1, 2 {
                          }
                          frame 3..5, Default {
                          }
                        }
                      }
                    }
                  }
                }
              }
              frame True {
                n947 = global read "G_rio.vi" "VS_CAN"() -> (w294:dbl)
                n948 = Absolute Value(x=w294) -> (abs(x)=w293:dbl)
                n949 = Less?(x=w293, y=0.05) -> (x < y?=w291:bool)
                n950 = global read "G_rio.vi" "Run"() -> (w296:bool)
                n951 = And(x=w291, y=w296) -> (x .and. y?=w295:bool)
                n952 = case shown="True" w295 {
                  tunnel: [_ w299] -> w297
                  frame False {
                  }
                  frame True {
                    n953 = local read "P, R, D"() -> (w298:i32)
                    n954 = case shown="-1" w298 {
                      tunnel: [w300 w305 w309] -> w299
                      frame -1 {
                        n955 = global read "G_rio.vi" "gear selector disp"() -> (w301:u8)
                        n956 = case shown="0" w301 {
                          tunnel: [-1.0 ("t") 1.0 ("t") _ _] -> w300
                          frame 0 {
                          }
                          frame 1, Default {
                          }
                          frame 4, 8 {
                          }
                          frame 7 {
                          }
                        }
                      }
                      frame 0, Default {
                        n957 = global read "G_rio.vi" "gear selector disp"() -> (w308:u8)
                        n958 = Equal To 0?(x=w308) -> (x = 0?=w307:bool)
                        n959 = Select(t=0.0, s=w307, f=1.0 ("t")) -> (s? t:f=w305:dbl)
                      }
                      frame 1 {
                        n960 = global read "G_rio.vi" "gear selector disp"() -> (w310:u8)
                        n961 = case shown="1, 2" w310 {
                          tunnel: [-1.0 1.0 0.0] -> w309
                          frame 0, 6, 7 {
                          }
                          frame 1, 2 {
                          }
                          frame 3..5, Default {
                          }
                        }
                      }
                    }
                  }
                }
              }
            }
            "shift lever" <- w262
          }
          frame #4 {
            n962 = flat-sequence {
              tunnel: [w331] -> w326
              tunnel: [w330] -> w325
              tunnel: [w327] -> w324
              tunnel: w326 -> [w493]
              tunnel: w325 -> [w495]
              tunnel: w324 -> [w494]
              frame #0 {
                n963 = global read "G_rio.vi" "Auto"() -> (w329:bool)
                n964 = flat-sequence {
                  tunnel: [w343] -> w332
                  frame #0 {
                    n965 = local read "Ref vel"() -> (w333:dbl)
                    n966 = global read "G_rio.vi" "accel pedal value"() -> (w335:dbl)
                    n967 = global read "G_rio.vi" "Throttle_Enable"() -> (w340:bool)
                    n968 = global read "G_rio.vi" "brake_act_can"() -> (w336:bool)
                    n969 = Not Equal To 0?(x=w333) -> (x != 0?=w342:bool)
                    n970 = Not(x=w336) -> (.not. x?=w341:bool)
                    n971 = Equal To 0?(x=w335) -> (x = 0?=w334:bool)
                    n972 = case shown="True" w334 {
                      tunnel: [TRUE w346] -> w337
                      frame False {
                        n973 = global write "G_rio.vi" "T lim counter 2"(u16 300 ("T lim counter 2")) -> ()
                      }
                      frame True {
                        n974 = global read "G_rio.vi" "T lim counter 2"() -> (w348:u16)
                        n975 = Decrement(x=w348) -> (x-1=w349:u16)
                        n976 = Max & Min(x=u16 0, y=w349) -> (max(x,y)=w347:u16)  [unwired: 1 out]
                        n977 = Not Equal To 0?(x=w347) -> (x != 0?=w346:bool)
                        n978 = global write "G_rio.vi" "T lim counter 2"(w347) -> ()
                      }
                    }
                    n979 = global read "G_rio.vi" "Auto"() -> (w338:bool)
                    n980 = global read "G_rio.vi" "Run"() -> (w339:bool)
                    n981 = Compound Arithmetic op=AND(w338, w339, w342, w341, w340, w337) -> (w343:bool)
                  }
                }
                n982 = case shown="True" w329 {
                  tunnel: [w379 w388] -> w328
                  frame False {
                    n983 = global read "G_rio.vi" "Brake Encoder mcp"() -> (w376:dbl)
                    n984 = global read "G_rio.vi" "brake encoder"() -> (w375:dbl)
                    n985 = Not Equal To 0?(x=w375) -> (x != 0?=w378:bool)
                    n986 = Subtract(x=0.0, y=w376) -> (x-y=w380:dbl)
                    n987 = Select(t=w380, s=w378, f=0.0) -> (s? t:f=w379:dbl)
                  }
                  frame True {
                    n988 = global read "G_rio.vi" "Run"() -> (w391:bool)
                    n989 = global read "G_rio.vi" "Brake Encoder mcp"() -> (w390:dbl)
                    n990 = case shown="True" w391 {
                      tunnel: [w392 w394] -> w386
                      frame False {
                        n991 = global read "G_rio.vi" "Ref Brk FULL"() -> (w392:dbl)
                      }
                      frame True {
                        n992 = local read "Ref vel"() -> (w393:dbl)
                        n993 = global read "G_rio.vi" "Ref Brk Enc"() -> (w397:dbl)
                        n994 = Equal To 0?(x=w393) -> (x = 0?=w398:bool)
                        n995 = global read "G_rio.vi" "Ref Brk FULL"() -> (w395:dbl)
                        n996 = Select(t=w395, s=w398, f=w397) -> (s? t:f=w396:dbl)
                        n997 = Max & Min(x=w395, y=w396) -> (min(x,y)=w394:dbl)  [unwired: 1 out]
                      }
                    }
                    n998 = global read "G_rio.vi" "brake encoder"() -> (w383:dbl)
                    n999 = Equal To 0?(x=w383) -> (x = 0?=w384:bool)
                    n1000 = Subtract(x=w386, y=w390) -> (x-y=w387:dbl)
                    n1001 = Equal To 0?(x=w386) -> (x = 0?=w385:bool)
                    n1002 = And(x=w384, y=w385) -> (x .and. y?=w382:bool)
                    n1003 = Select(t=0.0, s=w382, f=w387) -> (s? t:f=w388:dbl)
                  }
                }
                n1004 = flat-sequence {
                  tunnel: w328 -> [w361]
                  tunnel: [w356] -> w327
                  frame #0 {
                    n1005 = Multiply(x=w361, y=-0.01) -> (x*y=w363:dbl)
                    n1006 = In Range and Coerce(upper limit=1.0 ("x"), x=w363, lower limit=-1.0) -> (coerced(x)=w351:dbl)  [unwired: 1 out]
                    n1007 = flat-sequence {
                      tunnel: w351 -> [w369]
                      tunnel: [w370] -> w352
                      frame #0 {
                        w368 = 0.2 ("x")
                        n1008 = Multiply(x=w368, y=w369) -> (x*y=w367:dbl)
                        n1009 = Subtract(x=1.0, y=w368) -> (x-y=w373:dbl)
                        n1010 = feedback #16(0.0) -> (w371:dbl)
                        n1011 = Multiply(x=w371, y=w373) -> (x*y=w372:dbl)
                        n1012 = Add(x=w372, y=w367) -> (x+y=w370:dbl)
                        n1013 = feedback-in #16(w370) -> ()
                      }
                    }
                    n1014 = Multiply(x=w351, y=1.8 ("B P gain")) -> (x*y=w358:dbl)
                    n1015 = call "deadzone.vi"("min"=-15.0, "max"=15.0, "x"=w352) -> ("dead zone"=w353:dbl)  [unwired: 8 in]
                    n1016 = Multiply(x=w353, y=0.1 ("B D gain")) -> (x*y=w357:dbl)
                    n1017 = Add(x=w357, y=w358) -> (x+y=w356:dbl)
                  }
                }
                n1018 = case shown="True" w332 {
                  tunnel: [_ TRUE] -> w331
                  tunnel: [w399 w427] -> w330
                  frame False {
                    n1019 = flat-sequence {
                      tunnel: [w409] -> w399
                      frame #0 {
                        n1020 = global read "G_rio.vi" "T Lim"() -> (w400:bool)
                        n1021 = case shown="True" w400 {
                          selector: w400 -> [_ w407]
                          frame False {
                            n1022 = global write "G_rio.vi" "T lim counter"(u16 0 ("T lim counter")) -> ()
                          }
                          frame True {
                            n1023 = global write "G_rio.vi" "T lim once"(w407) -> ()
                            n1024 = global write "G_rio.vi" "T lim counter 2"(u16 300 ("T lim counter 2")) -> ()
                            n1025 = global read "G_rio.vi" "T lim counter"() -> (w406:u16)
                            n1026 = Increment(x=w406) -> (x+1=w405:u16)
                            n1027 = Max & Min(x=u16 100, y=w405) -> (min(x,y)=w404:u16)  [unwired: 1 out]
                            n1028 = global write "G_rio.vi" "T lim counter"(w404) -> ()
                          }
                        }
                      }
                      frame #1 {
                        n1029 = global read "G_rio.vi" "T lim once"() -> (w408:bool)
                        n1030 = case shown="True" w408 {
                          tunnel: [-1.0 ("t") w414] -> w409
                          frame False {
                          }
                          frame True {
                            n1031 = global read "G_rio.vi" "T lim counter"() -> (w413:u16)
                            n1032 = Equal?(x=w413, y=u16 100) -> (x = y?=w412:bool)
                            n1033 = Select(t=0.0, s=w412, f=-0.15) -> (s? t:f=w414:dbl)
                          }
                        }
                        n1034 = global write "G_rio.vi" "Throttle_Enable"(w408) -> ()
                      }
                    }
                  }
                  frame True {
                    n1035 = global write "G_rio.vi" "T lim counter"(u16 0 ("T lim counter")) -> ()
                    n1036 = global write "G_rio.vi" "T lim once"(FALSE ("T lim once")) -> ()
                    n1037 = global read "G_rio.vi" "Ref APS"() -> (w435:dbl)
                    n1038 = global read "G_rio.vi" "accel pedal value"() -> (w433:dbl)
                    n1039 = global read "G_rio.vi" "accel pedal value"() -> (w434:dbl)
                    n1040 = Subtract(x=w435, y=w434) -> (x-y=w428:dbl)
                    n1041 = Greater?(x=w433, y=95.0) -> (0:w419:bool)
                    n1042 = flat-sequence {
                      tunnel: w428 -> [w448]
                      tunnel: [w445] -> w426
                      frame #0 {
                        n1043 = feedback #17(0.0) -> (w453:dbl)
                        n1044 = feedback-in #17(w448) -> ()
                        n1045 = Multiply(x=w448, y=0.01) -> (x*y=w449:dbl)
                        n1046 = Subtract(x=w448, y=w453) -> (x-y=w452:dbl)
                        n1047 = feedback #18(0.0) -> (w444:dbl)
                        n1048 = Multiply(x=0.999, y=w444) -> (x*y=w443:dbl)
                        n1049 = Divide(x=w452, y=0.01) -> (x/y=w439:dbl)
                        n1050 = Add(x=w449, y=w443) -> (x+y=w440:dbl)
                        n1051 = feedback-in #18(w440) -> ()
                        n1052 = Build Array(w448, w440, w439) -> (w447:dbl[])
                        n1053 = Multiply(x=w447, y=dbl[] [8.0, 0.02, 0.5] ("pid gain 2")) -> (x*y=w446:dbl[])
                        n1054 = Add Array Elements(numeric array=w446) -> (sum=w445:dbl)
                      }
                    }
                    n1055 = Greater Than 0?(x=w428) -> (x > 0?=w418:bool)
                    n1056 = And(x=w419, y=w418) -> (x .and. y?=w430:bool)
                    n1057 = Multiply(x=w426, y=0.01) -> (x*y=w422:dbl)
                    n1058 = In Range and Coerce(upper limit=1.0 ("x"), x=w422, lower limit=-1.0) -> (coerced(x)=w425:dbl)  [unwired: 1 out]
                    n1059 = flat-sequence {
                      tunnel: w425 -> [w460]
                      tunnel: [w455] -> w424
                      frame #0 {
                        w461 = 0.5 ("x")
                        n1060 = Multiply(x=w461, y=w460) -> (x*y=w457:dbl)
                        n1061 = Subtract(x=1.0, y=w461) -> (x-y=w459:dbl)
                        n1062 = feedback #19(0.0) -> (w456:dbl)
                        n1063 = Multiply(x=w456, y=w459) -> (x*y=w458:dbl)
                        n1064 = Add(x=w458, y=w457) -> (x+y=w455:dbl)
                        n1065 = feedback-in #19(w455) -> ()
                      }
                    }
                    n1066 = Select(t=0.0 ("f"), s=w430, f=w424) -> (s? t:f=w427:dbl)
                  }
                }
              }
              frame #1 {
                n1067 = local read "shift lever"() -> (w465:dbl)
                n1068 = disable-structure shown="Enabled" {
                  disable-tunnel: [w496 _] -> w464
                  frame Disabled {
                    n1069 = global read "G_rio.vi" "Auto"() -> (w498:bool)
                    n1070 = global read "G_rio.vi" "Run"() -> (w497:bool)
                    n1071 = Compound Arithmetic op=AND(w498, w497) -> (w496:bool)
                  }
                  frame Enabled {
                  }
                }
                n1072 = Multiply(x=w494, y=600.0 ("B gain")) -> (x*y=w469:dbl)
                n1073 = Multiply(x=w495, y=500.0 ("T gain")) -> (x*y=w491:dbl)
                n1074 = local read "FPGA VI Reference Out"() -> (w474:refnum<k20>)
                n1075 = Multiply(x=w465, y=250.0 ("S gain")) -> (x*y=w476:dbl)
                n1076 = In Range and Coerce(upper limit=500.0, x=w491, lower limit=-500.0) -> (coerced(x)=w467:dbl)  [unwired: 1 out]
                n1077 = Select(t=w469, s="brake", f="Slide") -> (s? t:f=w471:dbl)
                n1078 = In Range and Coerce(upper limit=500.0, x=w476, lower limit=-500.0) -> (coerced(x)=w479:dbl)  [unwired: 1 out]
                n1079 = Add(x=w467, y=1500.0) -> (x+y=w487:dbl)
                n1080 = In Range and Coerce(upper limit=500.0, x=w471, lower limit=-500.0) -> (coerced(x)=w473:dbl)  [unwired: 1 out]
                n1081 = Add(x=w479, y=1500.0) -> (x+y=w481:dbl)
                n1082 = To Unsigned Word Integer(number=w487) -> (unsigned 16bit integer=w463:u16)
                "T PWM" <- w463
                n1083 = Add(x=w473, y=1500.0) -> (x+y=w486:dbl)
                n1084 = To Unsigned Word Integer(number=w481) -> (unsigned 16bit integer=w466:u16)
                n1085 = To Unsigned Word Integer(number=w486) -> (unsigned 16bit integer=w472:u16)
                "B PWM" <- w472
                n1086 = xnode "Read/Write Control"("FPGA VI Reference In"=w474, "Buzz"=w464, "S Pwm 1"=w466, "S Pwm 2"=w466, "B Pwm"=w472, "T Pwm"=w463, "Solenoid"=w493) -> ()  [unwired: 1 in, 2 out]
                "solenoid" <- w493
              }
              frame #2 {
                n1087 = local read "LCM"() -> (w499:bool)
                n1088 = case shown="True" w499 {
                  frame False {
                    n1089 = global read "G_rio.vi" "Auto"() -> (w500:bool)
                    n1090 = global read "G_rio.vi" "Run"() -> (w501:bool)
                    n1091 = global read "G_rio.vi" "VS_CAN"() -> (w503:dbl)
                    n1092 = shared-variable "veloster\\sharedvari.lvlib\\auto"(w500) -> ()  [unwired: 1 in, 1 out]
                    n1093 = shared-variable "veloster\\sharedvari.lvlib\\run"(w501) -> ()  [unwired: 1 in, 1 out]
                    n1094 = global read "G_rio.vi" "mdps str_ang"() -> (w502:dbl)
                    n1095 = shared-variable "veloster\\sharedvari.lvlib\\vs_can"(w503) -> ()  [unwired: 1 in, 1 out]
                    n1096 = shared-variable "veloster\\sharedvari.lvlib\\steer_output"(w502) -> ()  [unwired: 1 in, 1 out]
                  }
                  frame True {
                    n1097 = Get Date/Time In Seconds() -> (seconds since 1Jan1904=w508:timestamp)
                    n1098 = global read "G_rio.vi" "Ref Brk Enc"() -> (w511:dbl)
                    n1099 = local read "solenoid"() -> (w516:bool)
                    n1100 = local read "Ref steer"() -> (w509:dbl)
                    n1101 = global read "G_rio.vi" "Ref APS"() -> (w510:dbl)
                    n1102 = local read "brk enc"() -> (w515:u8)
                    n1103 = local read "B PWM"() -> (w514:u16)
                    n1104 = local read "T PWM"() -> (w513:u16)
                    n1105 = To Double Precision Float(number=w508) -> (double precision float=w507:dbl)
                    n1106 = global read "G_rio.vi" "LCM_CON_T"() -> (w527:T17)
                    n1107 = Unbundle By Name(w527) -> ("hash"=w525:i64)
                    n1108 = Multiply(x=w507, y=1000000.0) -> (x*y=w505:dbl)
                    n1109 = To Quad Integer(1:w505) -> (0:w504:i64)
                    n1110 = call "hash.vi"("input"=w525) -> ("output"=w524:i64)  [unwired: 10 in]
                    n1111 = local read "Ref vel"() -> (w512:dbl)
                    n1112 = global read "G_rio.vi" "T Lim"() -> (w517:bool)
                    n1113 = global read "G_rio.vi" "Auto"() -> (w519:bool)
                    n1114 = global read "G_rio.vi" "Run"() -> (w518:bool)
                    n1115 = Bundle(cluster=w527, "hash"=w524, "sys time"=w504, "Auto"=w519, "Run"=w518, "Solenoid"=w516, "T lim"=w517, "brk_enc"=w515, "B PWM"=w514, "T PWM"=w513, "ref_vel"=w512, "ref_bkr_enc"=w511, "ref_apv"=w510, "ref_steer"=w509) -> (w520:T17)
                    n1116 = Flatten To String(anything=w520, prepend array or string size? (T)=FALSE) -> (data string=w522:string)  [unwired: 2 in, 2 out]
                    n1117 = global read "G_rio.vi" "LCM"() -> (w521:T4)
                    n1118 = call "LCM_send.vi"("DATA"=w522, "ID"="CON_T", "LCM"=w521) -> ()  [unwired: 6 in, 3 out]
                  }
                }
              }
            }
          }
        }
      }
    }
  }
